vi "prius_all.vi"() -> ()   [LabVIEW 2015]
uses:
  <vilib>/Platform/TimedLoop/XDataNode/timing_clust.ctl
  <vilib>/Platform/TimedLoop/XDataNode/nitl_modes.ctl
  <vilib>/Platform/TimedLoop/XDataNode/wakeup.ctl
  <vilib>/myRIO/Instrument Drivers/Onboard IO/DIO/typedefs/DIO Reference.ctl
  <vilib>/myRIO/Common/Instrument Driver Framework/Utilities/typedefs/myRIO Generic Hardware Reference.ctl
  <vilib>/myRIO/Common/Instrument Driver Framework/Utilities/typedefs/Hardware Version Enum.ctl
  <vilib>/myRIO/Common/Instrument Driver Framework/Utilities/typedefs/myRIO v1.0 Reference.ctl
  <vilib>/myRIO/Common/Instrument Driver Framework/Utilities/typedefs/Generic FPGA Reference.ctl
  <vilib>/myRIO/Common/Instrument Driver Framework/myRIO v1.0/DIO/typedefs/DIO Channels List.ctl
  <vilib>/myRIO/Common/Instrument Driver Framework/myRIO v1.0/DIO/typedefs/DIO Channels Enum.ctl
  <vilib>/userdefined/High Color/nirio_resource_hc.ctl
  <vilib>/myRIO/Common/Instrument Driver Framework/myRIO v1.0/DIO/vis/myRIO v1.1 Open DIO.vi
  <vilib>/myRIO/Common/Instrument Driver Framework/Utilities/vis/Validate Channels.vi
  <vilib>/myRIO/Common/Instrument Driver Framework/myRIO v1.0/DIO/vis/myRIO v1.0 Reserve DIO.vi
  <vilib>/myRIO/Instrument Drivers/Onboard IO/PWM/vis/Set Duty Cycle and Frequency.vi
  <vilib>/myRIO/Common/Instrument Driver Framework/myRIO v1.0/DIO/vis/myRIO v1.0 Close DIO.vi
  <vilib>/myRIO/Common/Instrument Driver Framework/myRIO v1.0/AO/vis/myRIO v1.0 Close AO.vi
  <vilib>/myRIO/Common/Instrument Driver Framework/myRIO v1.0/PWM/vis/myRIO v1.0 Close PWM.vi
  <vilib>/myRIO/Common/Instrument Driver Framework/myRIO v1.0/Resource Manager/vis/myRIO v1.0 Reserve Channel List.vi
  <vilib>/myRIO/Common/Instrument Driver Framework/myRIO v1.0/DIO/vis/myRIO v1.0 Build MUX Configuration DIO.vi
  <vilib>/myRIO/Common/Instrument Driver Framework/myRIO v1.0/DIO/vis/myRIO v1.0 Unreserve DIO.vi
  <vilib>/myRIO/Common/Instrument Driver Framework/myRIO v1.0/AO/vis/myRIO v1.0 Unreserve AO.vi
  <vilib>/myRIO/Common/Instrument Driver Framework/myRIO v1.0/PWM/vis/myRIO v1.0 Unreserve PWM.vi
  <vilib>/myRIO/Common/Instrument Driver Framework/myRIO v1.0/Resource Manager/vis/myRIO v1.0 Reserve Channel.vi
  <vilib>/myRIO/Common/Instrument Driver Framework/myRIO v1.0/Resource Manager/vis/myRIO v1.0 Unreserve Channel.vi
  <vilib>/myRIO/Common/Instrument Driver Framework/myRIO v1.0/Resource Manager/vis/myRIO v1.0 Create Configuration List.vi
  <vilib>/myRIO/Common/Instrument Driver Framework/myRIO v1.0/Resource Manager/vis/myRIO v1.0 Unreserve Channel List.vi
  <vilib>/myRIO/Common/Instrument Driver Framework/myRIO v1.0/AO/vis/myRIO v1.0 Build MUX Configuration AO.vi
  <vilib>/myRIO/Common/Instrument Driver Framework/myRIO v1.0/PWM/vis/myRIO v1.0 Build MUX Configuration PWM.vi
  <vilib>/myRIO/Common/Instrument Driver Framework/myRIO v1.0/Resource Manager/vis/myRIO v1.0 Build Mutex Name.vi
  rio_Global.vi
  <vilib>/Utility/error.llb/Error Cluster From Error Code.vi
  <vilib>/myRIO/Common/Instrument Driver Framework/myRIO v1.0/PWM/vis/myRIO v1.0 Write PWM.vi
  <vilib>/Utility/VariantDataType/GetNumericInfo.vi
  <vilib>/myRIO/Common/Instrument Driver Framework/myRIO v1.0/myRIO v1.1 Open.vi
  <vilib>/myRIO/Common/Instrument Driver Framework/Utilities/vis/IO Manager.vi
  <vilib>/myRIO/Common/Instrument Driver Framework/Utilities/vis/Configuration Manager.vi
  <vilib>/myRIO/Common/Instrument Driver Framework/myRIO v1.0/Resource Manager/vis/myRIO v1.0 Configure IO.vi
  <vilib>/myRIO/Common/Instrument Driver Framework/myRIO v1.0/myRIO v1.0 Close.vi
  <vilib>/myRIO/Common/Instrument Driver Framework/myRIO v1.0/DIO/vis/myRIO v1.0 Write DIO.vi
  <vilib>/myRIO/Common/Instrument Driver Framework/myRIO v1.0/AO/vis/myRIO v1.0 Write AO.vi
  <vilib>/myRIO/Common/Instrument Driver Framework/myRIO v1.0/DIO/vis/myRIO v1.0 Shutdown DIO.vi
  <vilib>/myRIO/Common/Instrument Driver Framework/myRIO v1.0/PWM/vis/myRIO v1.0 Shutdown PWM.vi
  <vilib>/Analysis/Matrix/Numeric/Conversions/Array To Matrix - RA2.vi
  <vilib>/Analysis/Matrix/Numeric/Multiply/Multiply - RM,RM.vi
  <vilib>/Analysis/Matrix/Numeric/Add/Add - RM,RM.vi
  <vilib>/Analysis/baseanly.llb/Real Inverse Matrix.vi
  <vilib>/Analysis/Matrix/Numeric/Subtract/Subtract - RM,RM.vi
  <vilib>/Analysis/Matrix/Numeric/Conversions/Array To Matrix - RA.vi
  <vilib>/Analysis/Matrix/Numeric/Multiply/Multiply - R,RM.vi
  <vilib>/Analysis/Matrix/Numeric/Conversions/Matrix To Array - RM.vi
  <vilib>/myRIO/Instrument Drivers/Onboard IO/DIO/vis/myRIO DIO Open.xnode
  <vilib>/platform/TimedLoop/XDataNode/XDataNode.xnode
  <vilib>/myRIO/Instrument Drivers/Onboard IO/DIO/DIO.lvlib
  <vilib>/myRIO/Instrument Drivers/Onboard IO/PWM/PWM.lvlib
  <vilib>/myRIO/Instrument Drivers/Onboard IO/AO/AO.lvlib
  <vilib>/Analysis/Matrix/NI_Matrix.lvlib
  <vilib>/Analysis/NI_AALBase.lvlib
  <vilib>/Platform/TimedLoop/XDataNode/XDNodeRunTimeDep.lvlib
panel:
  in  "Ref_str_torque":dbl
  in  "invgain>1":dbl=4.499999999999998
  in  "mode":bool=TRUE
  in  "x":dbl
  out "Waveform Chart 2":dynamicdata(graph)=[{"t0"=timestamp(3543844041.358625 s since 1904-01-01), "dt"=1.0, "Y"=[0.015263023114702498]}, {"t0"=timestamp(3543844041.358625 s since 1904-01-01), "dt"=1.0, "Y"=[76.5]}]
  in  "x 2":dbl=0.002000000000000001 format="%#_13g"
  out "Ref_VS":dbl
  in  "y":dbl=0.003
  in  "min vel":i32=20
  in  "shift":dbl
  in  "lpf":dbl=0.8 format="%#_13g"
  in  "gain":dbl=0.79
  in  "str_gain":dbl=0.9 format="%#_13g"
  out "handle":dbl=-0.015263023114702498
  out "lane both":bool=TRUE
  out "get map name":bool
  out "map name":T1(ring)=enum."KAIST"
  in  "Steering Control":bool=TRUE
  out "fake_Ref_speed":dbl
  out "fake_Ref_str_ang":dbl
  out "Waveform Chart":dynamicdata(graph)=[{"t0"=timestamp(3543844041.358625 s since 1904-01-01), "dt"=1.0, "Y"=[0.015263023114702498]}, {"t0"=timestamp(3543844041.358625 s since 1904-01-01), "dt"=1.0, "Y"=[76.5]}]
  out "Gear":u8(ring) items=["P", "R", "N", "D"]
  out "read buffer":string="$GNGGA,114428.80,3623.46520,N,12724.00279,E,2,12,0.81,53.9,M,20.0,M,,0000*7B\r\n"
  out "yaw_rate":dbl=0.25
  out "XY Graph":cluster{"Y":dbl[], "Y":dbl[]}[](graph)=[{"Y"=[1.875, 1.875, 1.875, 1.875, 1.875, 1.875, 1.875, 1.875, 1.875, 1.875], "Y"=[0.0, 0.5, 1.0, 1.5, 2.0, 2.5, 3.0, 3.5, 4.0, 4.5]}, {"Y"=[-1.875, -1.875, -1.875, -1.875, -1.875, -1.875, -1.875, -1.875, -1.875, -1.875], "Y"=[0.0, 0.5, 1.0, 1.5, 2.0, 2.5, 3.0, 3.5, 4.0, 4.5]}, {"Y"=[-0.94, 0.94, 0.94, -0.94, -0.94], "Y"=[-3.2, -3.2, 1.5, 1.5, -3.2]}, {"Y"=[0.0, 0.0, 0.0, 0.0, 0.0, 0.0, 0.0, 0.0, 0.0, 0.0], "Y"=[0.0, 0.5, 1.0, 1.5, 2.0, 2.5, 3.0, 3.5, 4.0, 4.5]}, {"Y"=[-0.0, 0.002441079435136828, 0.009765016068527643, 0.021973905883363898, 0.03907124551911778, 0.061061937284492274, 0.08795229619902045, 0.11975005908698932, 0.15646439575426996, 0.19810592228603952, 0.2446867165104507, 0.2962203356814186, 0.3527218364413329, 0.41420779713322275, 0.48069634254055416, 0.5522071711422214, 0.6287615849803672, 0.7103825222489633, 0.7970945927225799, 0.8889241161567654, 0.9858991638044046, 1.0880496032065068, 1.1954071464308669, 1.3080054019486056, 1.4258799303560679, 1.5490683041691753, 1.677610171938241, 1.811547326954198, 1.950923780842551, 2.095785842368791, 2.246182201809347], "Y"=[0.0, 0.5, 1.0, 1.5, 2.0, 2.5, 3.0, 3.5, 4.0, 4.5, 5.0, 5.5, 6.0, 6.5, 7.0, 7.5, 8.0, 8.5, 9.0, 9.5, 10.0, 10.5, 11.0, 11.5, 12.0, 12.5, 13.0, 13.5, 14.0, 14.5, 15.0]}, {"Y"=[-0.0, 0.0008216505896712079, 0.0032866289850517205, 0.00739501506930651, 0.013146941995614725, 0.020542596208514396, 0.029582217474256822, 0.040266098919687465, 0.05259458707971021, 0.06656808195359076, 0.08218703706990027, 0.09945195956012753, 0.11836341024121566, 0.13892200370679575, 0.16112840842706078, 0.18498334685799023, 0.21048759555890229, 0.23764198531947045, 0.2664474012953235, 0.2969047831529963, 0.32901512522389, 0.3627794766672423, 0.39819894164267566, 0.4352746794916982, 0.474007904928726, 0.5143998882415417, 0.5564519555013874, 0.6001654887822383, 0.6455419263903934, 0.6925827631032746, 0.7412895504183155], "Y"=[0.0, 0.5, 1.0, 1.5, 2.0, 2.5, 3.0, 3.5, 4.0, 4.5, 5.0, 5.5, 6.0, 6.5, 7.0, 7.5, 8.0, 8.5, 9.0, 9.5, 10.0, 10.5, 11.0, 11.5, 12.0, 12.5, 13.0, 13.5, 14.0, 14.5, 15.0]}]
  out "Heading":dbl=-179.220077008385
  out "H_GPS":dbl
  out "pos":dbl[](array[numeric])=[1736.3543614568478, 3514.6262112945274]
  in  "GPS init":bool
  out "pos_gps":dbl[](array[numeric])=[42268800.0, 1.0, 1735.3231710957089, 3511.903145121578, -49.202530661854894, 42268800.0, 12.0, 18.0, 0.0, 0.81, 0.81, 0.0, 36.391086666666666, 127.4000465, 73.0] format="%#_19f"
  out "dt":dbl
  out "ecef ref":dbl[](array[numeric])=[-3119987.903302517, 4086549.99824973, 3761829.662354208]
  out "vgain":dbl=1.0353330715599283
  out "vcount":u64=227
  out "hbias":dbl=0.2579217148182668
  out "hcount":u64=1073
  out "get heading":bool
  out "get position":bool=TRUE
  out "heading error":dbl=3.127980429474107
  out "h_gps":dbl
  out "rt":dbl
  out "pos error":dbl=2.9758035193747063
  out "Kalmann init":bool
  out "VS_CAN":dbl
  out "car":refnum<k5>
  out "mdps str_ang":dbl=76.5
  out "eye":refnum<k5>
  out "APV":dbl
  out "PWM GAS":dbl=1000.0 min=1000.0 max=2000.0 step=1.0
  out "Auto":bool
  in  "Steering angle input":dbl(slide) min=-90.0 max=90.0 step=1.0 scale=-90.0..90.0
  in  "Steering angle input":bool=TRUE
  out "T init":i32=20
  out "T out":i32=20
  in  "manual speed":dbl
  in  "Velocity input":bool
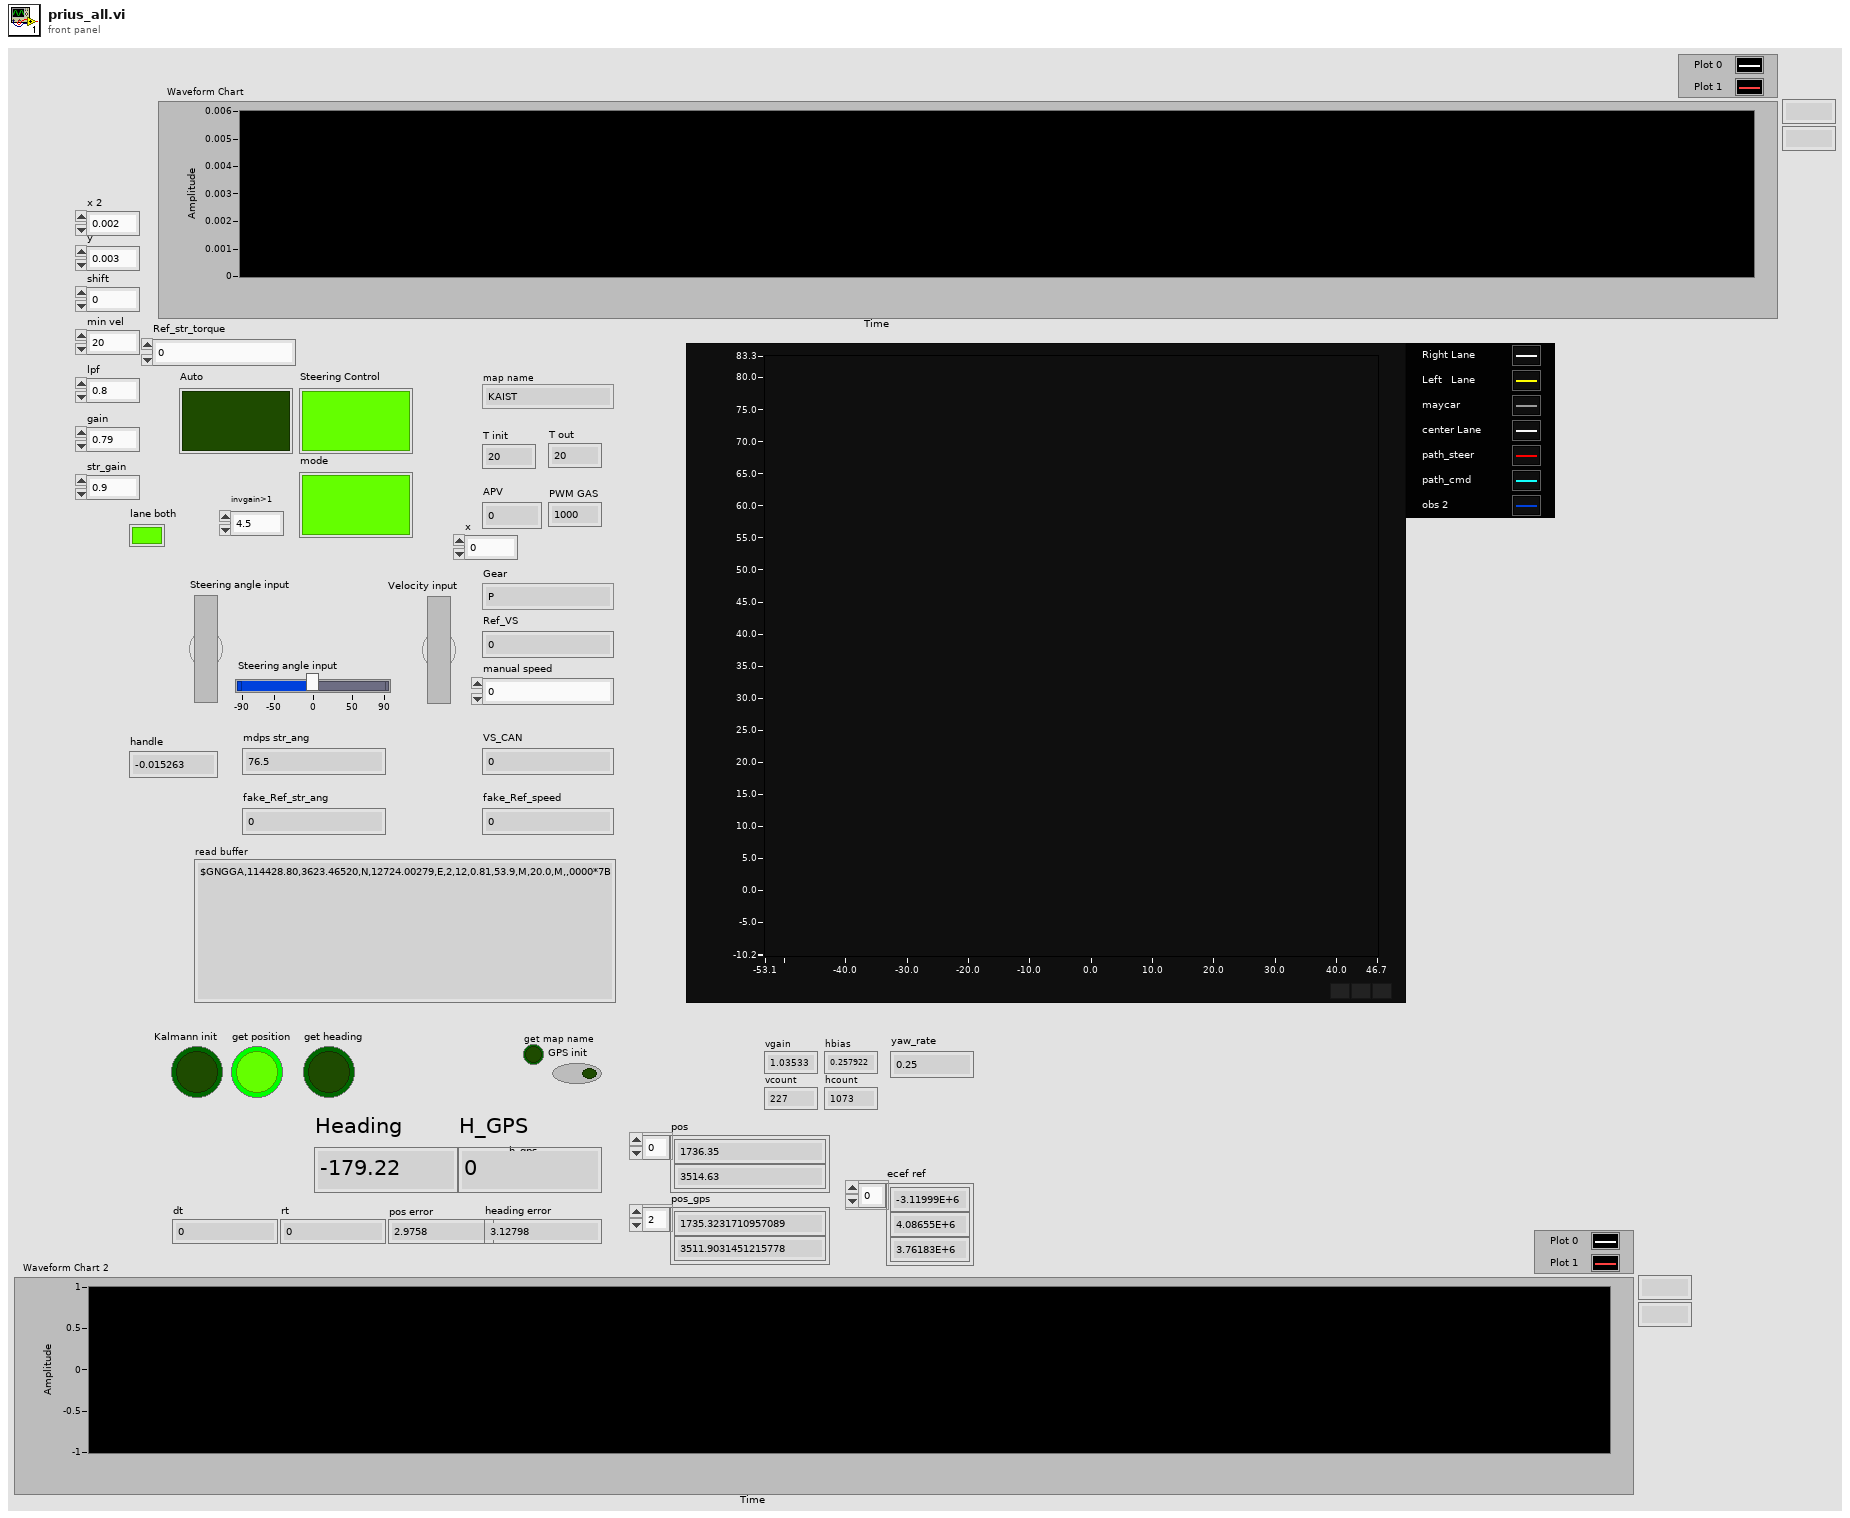
[diagram p1: front panel]
types:
  T1 = enum32{"Namyang", "Hyundai", "KAIST", "Ajou", "Munji", "Airforce", "Car", "KATRI", "Samsung", "Coex", "Gwangnaru"}
  T2 = typedef "XDNodeRunTimeDep.lvlib/timing_clust.ctl" = cluster{"Expected End [f-1]":u64, "Actual End [f-1]":u64, "Finished Late? [f-1]":bool, "Expected End [i-1]":u64, "Actual End [i-1]":u64, "Finished Late? [i-1]":bool, "Expected Start [i]":u64, "Actual Start [i]":u64, "Expected Start [f]":u64, "Actual Start [f]":u64, "Source Name":string, "Structure Name":string, "Period":i64, "Deadline":i64, "Offset":i64, "Start":i64, "Priority":i32, "Timeout":i32, "Mode":T3, "Wakeup Reason":T4, "Error":errorcluster, "Source Type":string, "Secondary Source Type":string, "Global End Time":u64, "Global Start Time":u64, "Frame Duration":u64, "Iteration Duration":u64, "Assigned CPU":i32, "I/O Scan Engine Mode":u32}
  T3 = typedef "XDNodeRunTimeDep.lvlib/nitl_modes.ctl" = enum32{"No Change", "Process missed periods, maintain original phase", "Discard missed periods, maintain original phase", "Process missed periods, ignore original phase", "Discard missed periods, ignore original phase"}
  T4 = typedef "XDNodeRunTimeDep.lvlib/wakeup.ctl" = enum32{"Normal", "Aborted", "Asynchronous wakeup", "Timing source error", "Timed loop error", "Timeout"}
  T5 = typedef "nirio_resource_hc.ctl" = tag
  T6 = typedef "Hardware Version Enum.ctl" = enum16{"Unknown", "myRIO-1900", "myRIO-1950", "roboRIO"}
  T7 = enum16{"Standard", "Buffered", "CRLF", "Immediate"}
  T8 = cluster{"identifier":u32, "timestamp":timestamp, "payload":u8[]}
  T9 = cluster{"connection ID":refnum<k16>, "net address":u32, "port":u16}
  T10 = cluster{"hash":i64, "sys time":i64, "size":i32, "data":u8[]}
  T11 = cluster{"hash":i64, "sys time":i64, "time":dbl, "yaw_rate":dbl, "mdps torque":dbl, "mdps str_ang":dbl, "VS_CAN":dbl, "lat_accel":dbl, "mcp":dbl, "accel pedal value":dbl, "tps":dbl, "odometer":dbl, "battery voltage":dbl, "WHL_SPD_RR":dbl, "WHL_SPD_RL":dbl, "WHL_SPD_FR":dbl, "WHL_SPD_FL":dbl}
  T12 = typedef "PWM.lvlib/PWM Reference.ctl" = cluster{"myRIO Reference":T13, "PWM Channels Enum":T16, "PWM Configuration":T17}
  T13 = typedef "myRIO Generic Hardware Reference.ctl" = cluster{"myRIO Model":T6, "myRIO Hardware Reference":T14}
  T14 = typedef "myRIO v1.0 Reference.ctl" = cluster{"Generic FPGA Reference":T15, "Allow multiple opens":bool}
  T15 = typedef "Generic FPGA Reference.ctl" = refnum<k20>
  T16 = typedef "PWM Channels Enum.ctl" = enum16{"Not Connected", "C/PWM0", "C/PWM1", "A/PWM0", "A/PWM1", "A/PWM2", "B/PWM0", "B/PWM1", "B/PWM2", "PWM/PWM0", "PWM/PWM1", "PWM/PWM2", "PWM/PWM3", "PWM/PWM4", "PWM/PWM5", "PWM/PWM6", "PWM/PWM7", "PWM/PWM8", "PWM/PWM9"}
  T17 = typedef "PWM.lvlib/PWM Configuration.ctl" = cluster{"Frequency":dbl, "Duty Cycle":dbl}
  T18 = typedef "AO.lvlib/AO Reference.ctl" = cluster{"myRIO Reference":T13, "AO Channel List":T19, "AO Scaling Constant List":T21}
  T19 = typedef "AO Channels List.ctl" = T20[]
  T20 = typedef "AO Channels Enum.ctl" = enum16{"Not Connected", "AudioOut/Left", "AudioOut/Right", "C/AO0", "C/AO1", "A/AO0", "A/AO1", "B/AO0", "B/AO1"}
  T21 = typedef "Analog Scaling Constants List.ctl" = T22[]
  T22 = typedef "Analog Scaling Constants.ctl" = cluster{"LSB Weight (Volts)":dbl, "Offset (Volts)":dbl, "Signed?":bool}
  T23 = typedef "DIO.lvlib/DIO Reference.ctl" = cluster{"myRIO Reference":T13, "DIO Channels List":T24}
  T24 = typedef "DIO Channels List.ctl" = T25[]
  T25 = typedef "DIO Channels Enum.ctl" = enum16{"Not Connected", "C/DIO0", "C/DIO1", "C/DIO2", "C/DIO3", "C/DIO4", "C/DIO5", "C/DIO6", "C/DIO7", "A/DIO0", "A/DIO1", "A/DIO2", "A/DIO3", "A/DIO4", "A/DIO5", "A/DIO6", "A/DIO7", "A/DIO8", "A/DIO9", "A/DIO10", "A/DIO11", "A/DIO12", "A/DIO13", "A/DIO14", "A/DIO15", "B/DIO0", "B/DIO1", "B/DIO2", "B/DIO3", "B/DIO4", "B/DIO5", "B/DIO6", "B/DIO7", "B/DIO8", "B/DIO9", "B/DIO10", "B/DIO11", "B/DIO12", "B/DIO13", "B/DIO14", "B/DIO15", "LED0", "LED1", "LED2", "LED3", "Button0", "DIO/DIO0", "DIO/DIO1", "DIO/DIO2", "DIO/DIO3", "DIO/DIO4", "DIO/DIO5", "DIO/DIO6", "DIO/DIO7", "DIO/DIO8", "DIO/DIO9", "SPI/CS0", "SPI/CS1", "SPI/CS2", "SPI/CS3", "LED RADIO (Green)", "LED RADIO (Red)", "LED COMM (Green)", "LED COMM (Red)", "LED MODE (Green)", "LED MODE (Red)"}
  T26 = cluster{"hash":i64, "sys time":i64, "ref_vel":dbl, "ref_steer":dbl, "alert":u8}
  T27 = cluster{"hash":i64, "sys time":i64, "ref_vel":dbl, "ref_steer":dbl}
  T28 = cluster{"hash":i64, "sys time":i64, "Auto":bool, "Run":bool, "Solenoid":bool, "T lim":bool, "brk_enc":u8, "B PWM":u16, "T PWM":u16, "ref_vel":dbl, "ref_bkr_enc":dbl, "ref_apv":dbl, "ref_steer":dbl}
  T29 = typedef "NI_Matrix.lvlib/RealMatrix.ctl" = dbl[][]
  T30 = cluster{"hash":i64, "sys time":i64, "dt":dbl, "x":dbl, "y":dbl, "speed":dbl, "heading":dbl, "yaw_rate":dbl}
  T31 = cluster{"Real 2D Array[0]":dbl, "Real 2D Array[1]":dbl, "Real 2D Array[2]":dbl, "Real 2D Array[3]":dbl, "Real 2D Array[4]":dbl}
  T32 = cluster{"hash":i64, "sys time":i64, "time":dbl, "x":dbl, "y":dbl, "h":dbl, "numSV":i32, "postype":i32, "lag":i32, "hordev":dbl, "lat":dbl, "lon":dbl, "hgt":dbl, "map_idx":i32}
  T33 = cluster{"output[0]":dbl, "output[1]":dbl, "output[2]":dbl, "output[3]":dbl, "output[4]":dbl, "output[5]":dbl, "output[6]":dbl, "output[7]":dbl, "output[8]":dbl, "output[9]":dbl, "output[10]":dbl, "output[11]":dbl, "output[12]":dbl, "output[13]":dbl, "output[14]":dbl}
  T34 = cluster{"hash":i64, "sys time":i64, "time":dbl, "speed":dbl, "heading":dbl, "lat":dbl, "lon":dbl}
  T35 = cluster{"output[0]":dbl, "output[1]":dbl, "output[2]":dbl, "output[3]":dbl, "output[4]":dbl, "output[5]":dbl, "output[6]":dbl}
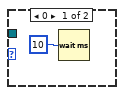
[diagram p2: hidden frame]
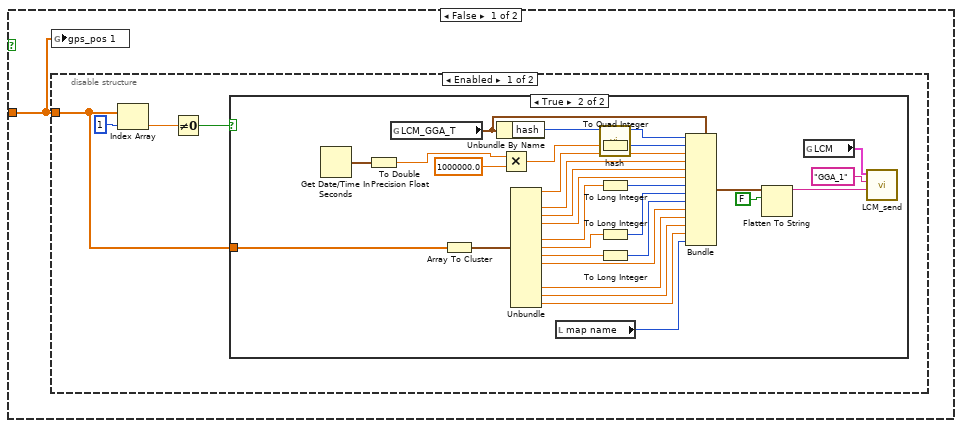
[diagram p4: hidden frame]
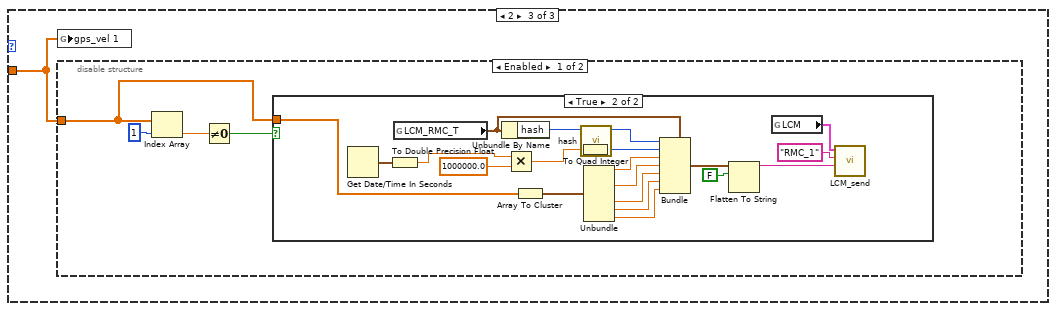
[diagram p7: hidden frame]
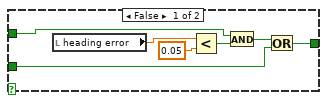
[diagram p13: hidden frame]
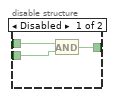
[diagram p14: hidden frame]
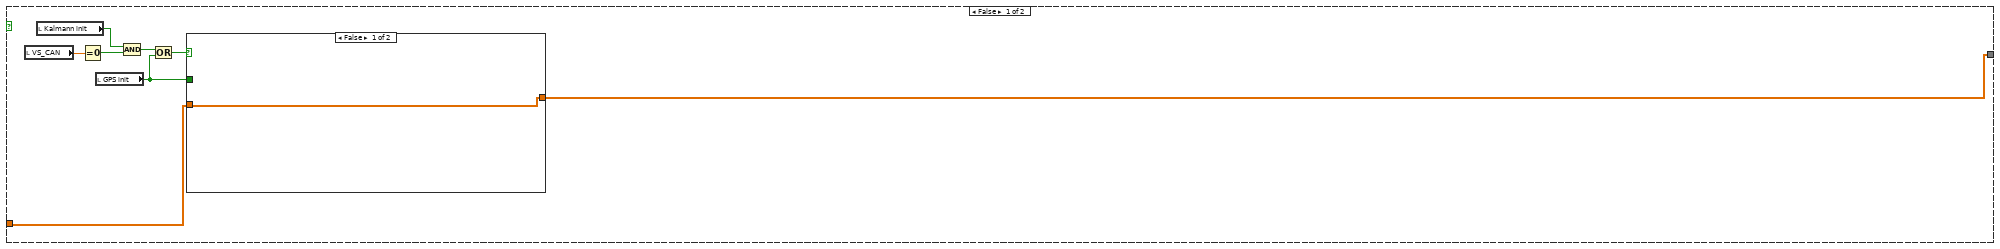
[diagram p15: hidden frame]
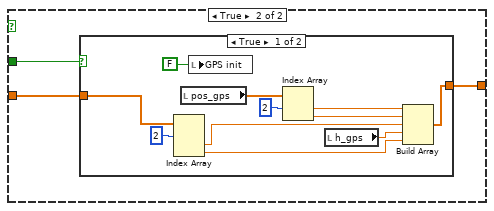
[diagram p16: hidden frame]
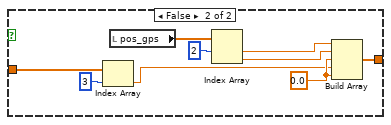
[diagram p17: hidden frame]
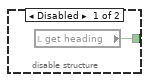
[diagram p19: hidden frame]
diagram:
  n1 = flat-sequence {
    frame #0 {
      w17 = u16 7668 ("port")
      w13 = u16 7665 ("port")
      n2 = disable-structure shown="Enabled" {
        frame Disabled {
        }
        frame Enabled {
          w36 = "Prius" ("Car_name")
          w37 = 0.0 ("Ref_str_ang")
          w38 = 1000.0 ("PWM GAS")
          w34 = FALSE ("Auto SW")
          n3 = global write "rio_Global.vi" "steering torque"(0.0 ("steering")) -> ()
          n4 = global write "rio_Global.vi" "Shift control"(0.0 ("Shift control")) -> ()
          n5 = global write "rio_Global.vi" "Solenoid"(FALSE ("CAN A 1")) -> ()
          n6 = global write "rio_Global.vi" "PWM GAS"(w38) -> ()
          n7 = global write "rio_Global.vi" "PWM Brake"(w38) -> ()
          n8 = global write "rio_Global.vi" "Ref_VS"(w37) -> ()
          n9 = global write "rio_Global.vi" "Ref_str_ang"(w37) -> ()
          n10 = global write "rio_Global.vi" "Auto"(w34) -> ()
          n11 = global write "rio_Global.vi" "Car_name"(w36) -> ()
          n12 = call "car_spec.vi"("Car_name"=w36) -> ("wheel base"=w31:dbl, "ratio"=w32:dbl, "overall width"=w33:dbl)  [unwired: 5 in, 3 out]
          n13 = global write "rio_Global.vi" "Auto SW"(w34) -> ()
          n14 = global write "rio_Global.vi" "ratio"(w32) -> ()
          n15 = global write "rio_Global.vi" "overall width"(w33) -> ()
          n16 = global write "rio_Global.vi" "wheel base"(w31) -> ()
        }
      }
      n17 = local read "eye"() -> (w19:refnum<k5>)
      n18 = local read "car"() -> (w20:refnum<k5>)
      n19 = global read "rio_Global.vi" "LCM PC"() -> (w10:T9)
      n20 = Equal?(x=refnum<k5> refnum ("connection ID"), y=w19) -> (x = y?=w21:bool)
      n21 = Equal?(x=refnum<k5> refnum ("connection ID"), y=w20) -> (x = y?=w23:bool)
      n22 = UDP Open(11:w17) -> (port=w15:refnum<k16>)  [unwired: 4 in, 2 out]
      n23 = Decrement(x=w13) -> (x-1=w12:u16)
      n24 = disable-structure shown="Enabled" {
        disable-tunnel: [w26 w29] -> w14
        disable-tunnel: w12 -> [w25 w30]
        frame Enabled {
          n25 = UDP Open(11:w25) -> (port=w26:refnum<k16>)  [unwired: 4 in, 2 out]
        }
        frame Disabled {
          n26 = String To IP(1:"239.255.76.67" ("name")) -> (0:w27:u32)
          n27 = UDP Multicast Open(10:w27, 11:w30) -> (3:w29:refnum<k16>)  [unwired: 3 in, 2 out]
        }
      }
      n28 = case shown="False" w21 {
        tunnel: w19 -> [w42 _]
        tunnel: [w41 w47] -> w18
        frame False {
          n29 = flat-sequence {
            tunnel: w42 -> [w43]
            tunnel: [w44] -> w41
            frame #0 {
              n30 = TCP Close Connection(connection ID=w43) -> ()  [unwired: 2 in, 2 out]
            }
            frame #1 {
              w45 = u16 3000  # port
              n31 = TCP Open Connection(address="192.168.0.100", remote port or service name=w45) -> (connection ID=w44:refnum<k5>)  [unwired: 3 in, 1 out]
            }
          }
        }
        frame True {
          w48 = u16 3000  # port
          n32 = TCP Open Connection(address="192.168.0.100", remote port or service name=w48) -> (connection ID=w47:refnum<k5>)  [unwired: 3 in, 1 out]
        }
      }
      "eye" <- w18
      n33 = case shown="False" w23 {
        tunnel: w20 -> [w51 _]
        tunnel: [w50 w56] -> w5
        frame False {
          n34 = flat-sequence {
            tunnel: w51 -> [w52]
            tunnel: [w53] -> w50
            frame #0 {
              n35 = TCP Close Connection(connection ID=w52) -> ()  [unwired: 2 in, 2 out]
            }
            frame #1 {
              w54 = u16 4000  # port
              n36 = TCP Open Connection(address="192.168.0.200", remote port or service name=w54) -> (connection ID=w53:refnum<k5>)  [unwired: 3 in, 1 out]
            }
          }
        }
        frame True {
          w57 = u16 4000  # port
          n37 = TCP Open Connection(address="192.168.0.200", remote port or service name=w57) -> (connection ID=w56:refnum<k5>)  [unwired: 3 in, 1 out]
        }
      }
      n38 = Bundle By Name(cluster=w10, "port"=w17, "connection ID"=w15, "net address"=u32 0) -> (w11:T9)
      n39 = global write "rio_Global.vi" "LCM PC"(w11) -> ()
      n40 = String To IP(1:"192.168.0.5" ("name")) -> (0:w2:u32)
      n41 = global read "rio_Global.vi" "LCM"() -> (w9:T9)
      n42 = Bundle By Name(cluster=w9, "port"=w13, "connection ID"=w14, "net address"=w2) -> (w8:T9)
      n43 = global write "rio_Global.vi" "LCM"(w8) -> ()
      n44 = TCP Read(connection ID=w5, bytes to read=999999, 9:1 ("timeout ms (25000)")) -> (connection ID out=→"car":refnum<k5>)  [unwired: 2 in, 2 out]
    }
    frame #1 {
      w87 = tag "B/PWM2"  # Brake
      w101 = tag[] ["B/AO0", "B/AO1"]  # Steering
      w108 = tag[] ["B/DIO4"]  # auto
      w111 = tag "B/PWM0"  # Accel
      w116 = tag[] ["B/DIO5", "B/DIO6"]  # Solenoid
      w78 = tag[] ["C/DIO7", "C/DIO6", "C/DIO5", "C/DIO0"]  # Shift X Eable
      w83 = tag[] ["C/AO0", "C/AO1"]  # Shift
      n45 = local read "eye"() -> (w92:refnum<k5>)
      n46 = local read "car"() -> (w88:refnum<k5>)
      n47 = while {
        tunnel: w92 -> [w302]
        tunnel: [w304] -> w95
        tunnel: [w303] -> w94
        shift-right: [w298] -> _
        shift-left: "" -> [w301]
        stop <- FALSE stop-if-true
        n48 = TCP Read(connection ID=w302, bytes to read=999999, 7:T7."Immediate" ("mode (standard)"), 9:1 ("timeout ms (25000)")) -> (connection ID out=w304:refnum<k5>, data out=w300:string, error out=w303:errorcluster)  [unwired: 1 in]
        n49 = Concatenate Strings(w301, w300) -> (w299:string)
        n50 = case shown="Default" w299 {
          selector: w299 -> [_ w312]
          tunnel: [_ w311] -> w298
          frame "" {
          }
          frame Default {
            n51 = flat-sequence {
              tunnel: w312 -> [w313]
              tunnel: [w314] -> w310
              tunnel: [w313] -> w309
              tunnel: [w343] -> w311
              tunnel: w310 -> [w343]
              tunnel: w309 -> [w342]
              frame #0 {
                n52 = while {
                  shift-right: [w321] -> w314
                  shift-left: w313 -> [w333]
                  stop <- w318 stop-if-true
                  w319 = "S" ("regular expression")
                  n53 = Match Pattern(string=w333, regular expression="S") -> (after substring=w331:string)  [unwired: 1 in, 3 out]
                  n54 = Match Pattern(string=w331, regular expression=" ") -> (before substring=w329:string, after substring=w326:string)  [unwired: 1 in, 2 out]
                  n55 = Hexadecimal String To Number(string=w329) -> (number=w316:u32)  [unwired: 2 in, 1 out]
                  n56 = Match Pattern(string=w326, regular expression=w319) -> (before substring=w325:string, match substring=w320:string, after substring=w322:string)  [unwired: 1 in, 1 out]
                  n57 = Not Equal?(x=w320, y=w319) -> (x != y?=w318:bool)
                  n58 = Concatenate Strings(w320, w322) -> (w321:string)
                  n59 = for {
                    N: 8 -> [_]
                    tunnel: w325 -> [w341]
                    tunnel: [w337] -> w315 mode=indexing
                    i -> [w336]
                    n60 = Multiply(x=2, y=w336) -> (x*y=w339:i32)
                    n61 = String Subset(string=w341, offset (0)=w339, length (rest)=2 ("length (rest)")) -> (substring=w334:string)
                    n62 = Hexadecimal String To Number(string=w334, default (0uL)=u8 0) -> (number=w337:u8)  [unwired: 1 in, 1 out]
                  }
                  n63 = Get Date/Time In Seconds() -> (seconds since 1Jan1904=w324:timestamp)
                  n64 = Bundle By Name(cluster=T8 {"identifier"=0, "timestamp"=timestamp(0 s since 1904-01-01), "payload"=[]} ("can cluster"), "identifier"=w316, "payload"=w315, "timestamp"=w324) -> (w323:T8)
                  n65 = call "mobileye_decoder.vi"("can cluster"=w323, "name"="Mobileye560") -> ()  [unwired: 10 in]
                }
              }
              frame #1 {
                n66 = disable-structure shown="Enabled" {
                  disable-tunnel: w342 -> [w345 _]
                  frame Enabled {
                    n67 = global read "rio_Global.vi" "LCM_CAN_RAW_SNAP"() -> (w358:T10)
                    n68 = Get Date/Time In Seconds() -> (seconds since 1Jan1904=w356:timestamp)
                    n69 = To Double Precision Float(number=w356) -> (double precision float=w355:dbl)
                    n70 = Unbundle By Name(w358) -> ("hash"=w353:i64)
                    n71 = Multiply(x=w355, y=1000000.0) -> (x*y=w357:dbl)
                    n72 = String To Byte Array(string=w345) -> (unsigned byte array=w346:u8[])
                    n73 = To Quad Integer(1:w357) -> (0:w348:i64)
                    n74 = call "hash.vi"("input"=w353) -> ("output"=w359:i64)  [unwired: 10 in]
                    n75 = Array Size(array=w346) -> (size(s)=w347:i32)
                    n76 = Bundle(cluster=w358, "hash"=w359, "sys time"=w348, "size"=w347, "data"=w346) -> (w351:T10)
                    n77 = Flatten To String(anything=w351, prepend array or string size? (T)=FALSE) -> (data string=w349:string)  [unwired: 2 in, 2 out]
                    n78 = global read "rio_Global.vi" "LCM"() -> (w350:T9)
                    n79 = call "LCM_send.vi"("DATA"=w349, "ID"="Mobileye560S", "LCM"=w350) -> ()  [unwired: 7 in, 2 out]
                  }
                  frame Disabled {
                  }
                }
              }
            }
          }
        }
      }
      n80 = while {
        tunnel: w88 -> [w209]
        tunnel: [w211] -> w89
        tunnel: [w210] -> w90
        shift-right: [w205] -> _
        shift-left: "" -> [w208]
        stop <- FALSE stop-if-true
        n81 = TCP Read(connection ID=w209, bytes to read=999999, 7:T7."Immediate" ("mode (standard)"), 9:1 ("timeout ms (25000)")) -> (connection ID out=w211:refnum<k5>, data out=w207:string, error out=w210:errorcluster)  [unwired: 1 in]
        n82 = Concatenate Strings(w208, w207) -> (w206:string)
        n83 = case shown="Default" w206 {
          selector: w206 -> [_ w219]
          tunnel: [_ w220] -> w205
          frame "" {
          }
          frame Default {
            n84 = flat-sequence {
              tunnel: w219 -> [w221]
              tunnel: [w222] -> w218
              tunnel: [w221] -> w217
              tunnel: w218 -> [w251]
              tunnel: w217 -> [w250]
              tunnel: [w251] -> w216
              tunnel: [w297] -> w220
              tunnel: w216 -> [w297]
              frame #0 {
                n85 = while {
                  shift-right: [w231] -> w222
                  shift-left: w221 -> [w241]
                  stop <- w228 stop-if-true
                  w229 = "S" ("regular expression")
                  n86 = Match Pattern(string=w241, regular expression="S") -> (after substring=w239:string)  [unwired: 1 in, 3 out]
                  n87 = Match Pattern(string=w239, regular expression=" ") -> (before substring=w237:string, after substring=w235:string)  [unwired: 1 in, 2 out]
                  n88 = Hexadecimal String To Number(string=w237) -> (number=w226:u32)  [unwired: 2 in, 1 out]
                  n89 = Match Pattern(string=w235, regular expression=w229) -> (before substring=w234:string, match substring=w230:string, after substring=w232:string)  [unwired: 1 in, 1 out]
                  n90 = Not Equal?(x=w230, y=w229) -> (x != y?=w228:bool)
                  n91 = Concatenate Strings(w230, w232) -> (w231:string)
                  n92 = for {
                    N: 8 -> [_]
                    tunnel: w234 -> [w249]
                    tunnel: [w245] -> w225 mode=indexing
                    i -> [w244]
                    n93 = Multiply(x=2, y=w244) -> (x*y=w247:i32)
                    n94 = String Subset(string=w249, offset (0)=w247, length (rest)=2 ("length (rest)")) -> (substring=w242:string)
                    n95 = Hexadecimal String To Number(string=w242, default (0uL)=u8 0) -> (number=w245:u8)  [unwired: 1 in, 1 out]
                  }
                  n96 = Get Date/Time In Seconds() -> (seconds since 1Jan1904=w233:timestamp)
                  n97 = Bundle By Name(cluster=T8 {"identifier"=0, "timestamp"=timestamp(0 s since 1904-01-01), "payload"=[]} ("can cluster"), "identifier"=w226, "payload"=w225, "timestamp"=w233) -> (w223:T8)
                  n98 = global read "rio_Global.vi" "Car_name"() -> (w224:string)
                  n99 = call "can decoder.vi"("can cluster"=w223, "name"=w224) -> ()  [unwired: 10 in]
                }
              }
              frame #1 {
                n100 = disable-structure shown="Enabled" {
                  disable-tunnel: w250 -> [w252 _]
                  frame Enabled {
                    n101 = global read "rio_Global.vi" "LCM_CAN_RAW_SNAP"() -> (w254:T10)
                    n102 = Get Date/Time In Seconds() -> (seconds since 1Jan1904=w256:timestamp)
                    n103 = To Double Precision Float(number=w256) -> (double precision float=w257:dbl)
                    n104 = Unbundle By Name(w254) -> ("hash"=w259:i64)
                    n105 = Multiply(x=w257, y=1000000.0) -> (x*y=w255:dbl)
                    n106 = String To Byte Array(string=w252) -> (unsigned byte array=w267:u8[])
                    n107 = To Quad Integer(1:w255) -> (0:w265:i64)
                    n108 = call "hash.vi"("input"=w259) -> ("output"=w253:i64)  [unwired: 10 in]
                    n109 = Array Size(array=w267) -> (size(s)=w266:i32)
                    n110 = Bundle(cluster=w254, "hash"=w253, "sys time"=w265, "size"=w266, "data"=w267) -> (w261:T10)
                    n111 = global read "rio_Global.vi" "Car_name"() -> (w264:string)
                    n112 = Flatten To String(anything=w261, prepend array or string size? (T)=FALSE) -> (data string=w263:string)  [unwired: 2 in, 2 out]
                    n113 = global read "rio_Global.vi" "LCM"() -> (w262:T9)
                    n114 = call "LCM_send.vi"("DATA"=w263, "ID"=w264, "LCM"=w262) -> ()  [unwired: 7 in, 2 out]
                  }
                  frame Disabled {
                  }
                }
              }
              frame #2 {
                n115 = Get Date/Time In Seconds() -> (seconds since 1Jan1904=w288:timestamp)
                n116 = global read "rio_Global.vi" "LCM_CAN_T"() -> (w270:T11)
                n117 = To Double Precision Float(number=w288) -> (double precision float=w289:dbl)
                n118 = global read "rio_Global.vi" "C_mdps str_ang"() -> (w269:dbl)
                n119 = global read "rio_Global.vi" "C_battery voltage"() -> (w273:dbl)
                n120 = global read "rio_Global.vi" "C_WHL_SPD_RR"() -> (w274:dbl)
                n121 = global read "rio_Global.vi" "C_WHL_SPD_RL"() -> (w275:dbl)
                n122 = global read "rio_Global.vi" "C_WHL_SPD_FR"() -> (w271:dbl)
                n123 = global read "rio_Global.vi" "C_WHL_SPD_FL"() -> (w276:dbl)
                n124 = global read "rio_Global.vi" "C_mdps torque"() -> (w283:dbl)
                n125 = Unbundle By Name(w270) -> ("hash"=w291:i64)
                n126 = Multiply(x=w289, y=1000000.0) -> (x*y=w287:dbl)
                n127 = global read "rio_Global.vi" "C_odometer"() -> (w277:dbl)
                n128 = global read "rio_Global.vi" "C_yaw_rate"() -> (w284:dbl)
                n129 = global read "rio_Global.vi" "C_VS_CAN"() -> (w282:dbl)
                n130 = global read "rio_Global.vi" "C_MCP"() -> (w280:dbl)
                n131 = global read "rio_Global.vi" "C_APV"() -> (w279:dbl)
                n132 = To Quad Integer(1:w287) -> (0:w296:i64)
                n133 = Negate(x=w269) -> (-x=w268:dbl)
                n134 = call "hash.vi"("input"=w291) -> ("output"=w286:i64)  [unwired: 10 in]
                n135 = global read "rio_Global.vi" "time"() -> (w285:dbl)
                n136 = Bundle(cluster=w270, "hash"=w286, "sys time"=w296, "time"=w285, "yaw_rate"=w284, "mdps torque"=w283, "mdps str_ang"=w268, "VS_CAN"=w282, "lat_accel"=0.0, "mcp"=w280, "accel pedal value"=w279, "tps"=0.0, "odometer"=w277, "battery voltage"=w273, "WHL_SPD_RR"=w274, "WHL_SPD_RL"=w275, "WHL_SPD_FR"=w271, "WHL_SPD_FL"=w276) -> (w293:T11)
                n137 = Flatten To String(anything=w293, prepend array or string size? (T)=FALSE) -> (data string=w295:string)  [unwired: 2 in, 2 out]
                n138 = global read "rio_Global.vi" "LCM"() -> (w294:T9)
                n139 = call "LCM_send.vi"("DATA"=w295, "ID"="CAN_T", "LCM"=w294) -> ()  [unwired: 7 in, 2 out]
              }
            }
          }
        }
      }
      n140 = call <vilib>:"Smart Open.vi"("Allow multiple opens?"=FALSE, "Channel Name"=w87) -> ("error out"=w61:errorcluster, "PWM Ref Out"=w64:T12)  [unwired: 8 in]
      n141 = call <vilib>:"Smart Open.vi"("Allow multiple opens?"=FALSE, "Channel Name"=w111) -> ("error out"=w69:errorcluster, "PWM Ref Out"=w68:T12)  [unwired: 8 in]
      n142 = call <vilib>:"Set Frequency.vi"("error in (no error)"=w61, "Frequency [Hz]"=50.0, "PWM Ref In"=w64) -> ("error out"=w60:errorcluster, "PWM Ref Out"=w63:T12)  [unwired: 6 in]
      n143 = call <vilib>:"Set Frequency.vi"("error in (no error)"=w69, "Frequency [Hz]"=50.0, "PWM Ref In"=w68) -> ("error out"=w66:errorcluster, "PWM Ref Out"=w67:T12)  [unwired: 6 in]
      n144 = call <vilib>:"Smart Open.vi"("Allow multiple opens?"=TRUE, "Channel Names"=w101) -> ("error out"=w99:errorcluster, "AO Ref Out"=w100:T18)  [unwired: 8 in]
      n145 = call <vilib>:"Smart Open.vi"("Allow multiple opens?"=FALSE, "Channel Names"=w108) -> ("error out"=w106:errorcluster, "DIO Ref Out"=w107:T23)  [unwired: 8 in]
      n146 = xnode "myRIO DIO Open.xnode"("Allow multiple opens?"=TRUE, "Channel Names"=w116) -> ("error out"=w114:errorcluster, "DIO Ref Out"=w115:T23)  [unwired: 1 in]
      n147 = xnode "myRIO DIO Open.xnode"("Allow multiple opens?"=TRUE, "Channel Names"=w78) -> ("error out"=w73:errorcluster, "DIO Ref Out"=w76:T23)  [unwired: 1 in]
      n148 = call <vilib>:"Smart Open.vi"("Allow multiple opens?"=TRUE, "Channel Names"=w83) -> ("error out"=w79:errorcluster, "AO Ref Out"=w82:T18)  [unwired: 8 in]
      n149 = node-c288(i64 10 ("Period")) -> (w72:T2)  [unwired: 3 in]
      n150 = timed-loop {
        tunnel: w115 -> [w181]
        tunnel: [w182] -> w113
        tunnel: w114 -> [w180]
        tunnel: [w176] -> w112
        tunnel: w107 -> [w174]
        tunnel: [w174] -> w105
        tunnel: w106 -> [w173]
        tunnel: [w173] -> w104
        tunnel: w100 -> [w172]
        tunnel: [w170] -> w98
        tunnel: w99 -> [w171]
        tunnel: [w169] -> w97
        tunnel: w67 -> [w178]
        tunnel: [w179] -> w110
        tunnel: w66 -> [w177]
        tunnel: [w175] -> w109
        tunnel: w63 -> [w167]
        tunnel: [w166] -> w85
        tunnel: w82 -> [w165]
        tunnel: [w164] -> w81
        tunnel: [w163] -> w80
        tunnel: w79 -> [w162]
        tunnel: w76 -> [w161]
        tunnel: [w160] -> w75
        tunnel: [w159] -> w74
        tunnel: w73 -> [w158]
        timing: w72 -> [_]
        timing-out: [_] -> w71
        tunnel: w60 -> [w128]
        tunnel: [w127] -> w59
        stop <- FALSE ("Auto") stop-if-true
        w148 = 0.0 ("y")
        n151 = node-c288() -> ()  [unwired: 1 in]
        n152 = global read "rio_Global.vi" "PWM Brake"() -> (w120:dbl)
        n153 = global read "rio_Global.vi" "PWM GAS"() -> (w123:dbl)
        n154 = global read "rio_Global.vi" "Solenoid"() -> (w121:bool)
        n155 = global read "rio_Global.vi" "steering torque"() -> (w144:dbl)
        n156 = global read "rio_Global.vi" "Shift control"() -> (w132:dbl)
        n157 = global read "rio_Global.vi" "C_VS_CAN"() -> (w140:dbl)
        n158 = global read "rio_Global.vi" "Auto"() -> (w119:bool)
        n159 = global read "rio_Global.vi" "Auto"() -> (w124:bool)
        n160 = global read "rio_Global.vi" "Auto"() -> (w122:bool)
        n161 = Select(t=w121, s=w122, f=w122) -> (s? t:f=w126:bool)
        n162 = Negate(x=w144) -> (-x=w146:dbl)
        n163 = Equal To 0?(x=w140) -> (x = 0?=w130:bool)
        n164 = Not Equal To 0?(x=w132) -> (x != 0?=w131:bool)
        n165 = Select(t=w120, s=w119, f=1000.0) -> (s? t:f=w142:dbl)
        n166 = Select(t=w123, s=w124, f=1000.0) -> (s? t:f=w147:dbl)
        n167 = global read "rio_Global.vi" "Auto"() -> (w145:bool)
        n168 = global read "rio_Global.vi" "Auto"() -> (w141:bool)
        n169 = Build Array(w126, w126) -> (w152:bool[])
        n170 = Select(t=w146, s=w145, f=w148) -> (s? t:f=w149:dbl)
        n171 = call <vilib>:"Write.vi"("error in (no error)"=w180, "Values"=w152, "DIO Ref In"=w181) -> ("error out"=w176:errorcluster, "DIO Ref Out"=w182:T23)  [unwired: 6 in]
        n172 = Compound Arithmetic op=AND(w130, w141, w131) -> (w137:bool)
        n173 = Divide(x=w142, y=20000.0) -> (x/y=w129:dbl)
        n174 = Divide(x=w147, y=20000.0) -> (x/y=w150:dbl)
        n175 = Max & Min(x=w149, y=w148) -> (min(x,y)=w154:dbl)  [unwired: 1 out]
        n176 = Select(t=w132, s=w137, f=0.0 ("element")) -> (s? t:f=w134:dbl)
        n177 = Build Array(w137, w137, w137, FALSE ("element")) -> (w139:bool[])
        n178 = call <vilib>:"Write.vi"("error in (no error)"=w158, "Values"=w139, "DIO Ref In"=w161) -> ("error out"=w159:errorcluster, "DIO Ref Out"=w160:T23)  [unwired: 6 in]
        n179 = Negate(x=w154) -> (-x=w153:dbl)
        n180 = call <vilib>:"Set Duty Cycle.vi"("error in (no error)"=w128, "Duty Cycle"=w129, "PWM Ref In"=w167) -> ("error out"=w127:errorcluster, "PWM Ref Out"=w166:T12)  [unwired: 6 in]
        n181 = call <vilib>:"Set Duty Cycle.vi"("error in (no error)"=w177, "Duty Cycle"=w150, "PWM Ref In"=w178) -> ("error out"=w175:errorcluster, "PWM Ref Out"=w179:T12)  [unwired: 6 in]
        n182 = Max & Min(x=0.0, y=w149) -> (max(x,y)=w155:dbl)  [unwired: 1 out]
        n183 = Build Array(0.0 ("element"), w134) -> (w133:dbl[])
        n184 = call <vilib>:"Write.vi"("error in (no error)"=w162, "Values"=w133, "AO Ref In"=w165) -> ("error out"=w163:errorcluster, "AO Ref Out"=w164:T18)  [unwired: 6 in]
        n185 = Build Array(w155, w153) -> (w157:dbl[])
        n186 = call <vilib>:"Write.vi"("error in (no error)"=w171, "Values"=w157, "AO Ref In"=w172) -> ("error out"=w169:errorcluster, "AO Ref Out"=w170:T18)  [unwired: 6 in]
        n187 = node-c288() -> ()  [unwired: 1 out]
      }
      n188 = node-c288(w71) -> ()  [unwired: 1 out]
      n189 = call <vilib>:"Close.vi"("error in (no error)"=w97, "AO Ref In"=w98) -> ()  [unwired: 9 in, 1 out]
      n190 = call <vilib>:"Close.vi"("error in (no error)"=w59, "PWM Ref In"=w85) -> ()  [unwired: 9 in, 1 out]
      n191 = call <vilib>:"Close.vi"("error in (no error)"=w104, "DIO Ref In"=w105) -> ()  [unwired: 9 in, 1 out]
      n192 = call <vilib>:"Close.vi"("error in (no error)"=w109, "PWM Ref In"=w110) -> ()  [unwired: 9 in, 1 out]
      n193 = call <vilib>:"Close.vi"("error in (no error)"=w112, "DIO Ref In"=w113) -> ()  [unwired: 9 in, 1 out]
      n194 = call <vilib>:"Close.vi"("error in (no error)"=w74, "DIO Ref In"=w75) -> ()  [unwired: 9 in, 1 out]
      n195 = call <vilib>:"Close.vi"("error in (no error)"=w80, "AO Ref In"=w81) -> ()  [unwired: 9 in, 1 out]
      n196 = TCP Close Connection(connection ID=w95, error in (no error)=w94) -> ()  [unwired: 1 in, 2 out]
      n197 = TCP Close Connection(connection ID=w89, error in (no error)=w90) -> ()  [unwired: 1 in, 2 out]
    }
  }
  n198 = flat-sequence {
    frame #0 {
      w380 = 0.0 ("fake_Ref_str_ang")
      w379 = FALSE ("Velocity input")
      n199 = local write "manual speed"(0.0 ("manual speed")) -> ()
      n200 = local write "Steering angle input"(0.0 ("con_vs")) -> ()
      n201 = local write "mode"(FALSE ("mode")) -> ()
      n202 = local write "Steering angle input"(FALSE ("Steering torque input")) -> ()
      n203 = global write "rio_Global.vi" "lane width"(3.5 ("lane width")) -> ()
      n204 = local write "Velocity input"(w379) -> ()
      n205 = local write "Steering Control"(w379) -> ()
      "fake_Ref_str_ang" <- w380
      "fake_Ref_speed" <- w380
      "lane both" <- FALSE ("lane both")
    }
    frame #1 {
      n206 = while {
        stop <- FALSE stop-if-true
        n207 = flat-sequence {
          tunnel: [w694] -> w384
          tunnel: w384 -> [w723]
          frame #0 {
            n208 = Wait Until Next ms Multiple(millisecond multiple=u32 10) -> ()  [unwired: 1 out]
          }
          frame #1 {
            n209 = disable-structure shown="Disabled" {
              disable-tunnel: [w390 "Mobileye" ("ID")] -> w388
              disable-tunnel: [w389 _] -> w387
              frame Enabled {
                n210 = global read "rio_Global.vi" "LCM PC"() -> (w391:T9)
                n211 = call "LCM_read.vi"("LCM"=w391) -> ("data"=w389:string, "ID"=w390:string)  [unwired: 7 in, 2 out]
              }
              frame Disabled {
              }
            }
            n212 = case shown="\"Mobileye\"" w388 {
              tunnel: w387 -> [_ _ w677]
              frame "Mobileye" {
                n213 = flat-sequence {
                  frame #0 {
                    w411 = 2 ("index")
                    w415 = 2 ("index")
                    n214 = global read "rio_Global.vi" "C_VS_CAN"() -> (w400:dbl)
                    n215 = global read "rio_Global.vi" "M_lane_right"() -> (w408:dbl[])
                    n216 = global read "rio_Global.vi" "M_headway"() -> (w394:dbl)
                    n217 = global read "rio_Global.vi" "M_lane_left"() -> (w407:dbl[])
                    n218 = Divide(x=w400, y=3.6) -> (x/y=w398:dbl)
                    n219 = Multiply(x=w398, y=w394) -> (x*y=w397:dbl)
                    n220 = Index Array(array=w407, index=w415) -> (element=w414:dbl)
                    n221 = Index Array(array=w408, index=w411) -> (element=w412:dbl)
                    n222 = Greater Or Equal?(x=w414, y=w415) -> (x >= y?=w413:bool)
                    n223 = Greater Or Equal?(x=w412, y=w411) -> (x >= y?=w410:bool)
                    n224 = Multiply(x=w397, y=2.0) -> (x*y=w396:dbl)
                    n225 = local read "lane both"() -> (w418:bool)
                    n226 = Or(x=w413, y=w410) -> (x .or. y?=w419:bool)
                    n227 = And(x=w413, y=w410) -> (x .and. y?=w417:bool)
                    n228 = Not Equal To 0?(x=w394) -> (x != 0?=w393:bool)
                    n229 = And(x=w419, y=w418) -> (x .and. y?=w416:bool)
                    n230 = Max & Min(x="x", y=w396) -> (min(x,y)=w401:dbl)  [unwired: 1 out]
                    n231 = case shown="True" w393 {
                      tunnel: w401 -> [_ w422]
                      frame False {
                      }
                      frame True {
                        n232 = global write "rio_Global.vi" "Ref_VS"(w422) -> ()
                      }
                    }
                    n233 = Or(x=w417, y=w416) -> (x .or. y?=w409:bool)
                    n234 = case shown="True" w409 {
                      tunnel: w407 -> [_ w426]
                      tunnel: w408 -> [_ w424]
                      tunnel: [_ w430] -> w420
                      frame False {
                        n235 = local write "lane both"(FALSE ("lane both")) -> ()
                      }
                      frame True {
                        w428 = 2 ("index")
                        w433 = 2 ("index")
                        n236 = Index Array(array=w426, index=w433) -> (element=w432:dbl)
                        n237 = Index Array(array=w424, index=w428) -> (element=w429:dbl)
                        n238 = Greater Or Equal?(x=w429, y=w428) -> (x >= y?=w425:bool)
                        n239 = Greater Or Equal?(x=w432, y=w433) -> (x >= y?=w427:bool)
                        n240 = And(x=w427, y=w425) -> (x .and. y?=w431:bool)
                        n241 = case shown="False" w431 {
                          tunnel: w426 -> [w455 w457]
                          tunnel: w424 -> [w450 w456]
                          tunnel: [w448 w464] -> w430
                          tunnel: w427 -> [w434 _]
                          frame False {
                            w443 = 0.2 ("y")
                            w446 = 5 ("index")
                            w454 = 5 ("index")
                            n242 = global read "rio_Global.vi" "overall width"() -> (w436:dbl)
                            n243 = Index Array(array=w455, index=w454) -> (element=w452:dbl)
                            n244 = Index Array(array=w450, index=w446) -> (element=w445:dbl)
                            n245 = global read "rio_Global.vi" "lane width"() -> (w435:dbl)
                            n246 = Multiply(x=w436, y=w443) -> (x*y=w441:dbl)
                            n247 = Add(x=w441, y=w443) -> (x+y=w437:dbl)
                            n248 = Add(x=1.0 ("y"), y=w441) -> (x+y=w438:dbl)
                            n249 = Multiply(x=w435, y=0.5) -> (x*y=w440:dbl)
                            n250 = In Range and Coerce(upper limit=w438, x=w440, lower limit=w437) -> (coerced(x)=w439:dbl)  [unwired: 1 out]
                            n251 = Add(x=w452, y=w439) -> (x+y=w451:dbl)
                            n252 = Subtract(x=w445, y=w439) -> (x-y=w444:dbl)
                            n253 = Replace Array Subset(array=w455, new element=w451, index=w454) -> (w449:dbl[])
                            n254 = Replace Array Subset(array=w450, new element=w444, index=w446) -> (w447:dbl[])
                            n255 = Select(t=w449, s=w434, f=w447) -> (s? t:f=w448:dbl[])
                          }
                          frame True {
                            n256 = Add(x=w457, y=w456) -> (x+y=w466:dbl[])
                            n257 = Index Array(array=w456, index=5) -> (element=w462:dbl)
                            n258 = Index Array(array=w457, index=5) -> (element=w459:dbl)
                            n259 = local write "lane both"(TRUE ("lane both")) -> ()
                            n260 = Subtract(x=w462, y=w459) -> (x-y=w458:dbl)
                            n261 = global write "rio_Global.vi" "lane width"(w458) -> ()
                            n262 = Multiply(x=0.5, y=w466) -> (x*y=w464:dbl[])
                          }
                        }
                      }
                    }
                    n263 = Empty Array?(array=w420) -> (empty?=w421:bool)
                    n264 = global write "rio_Global.vi" "M_lane_center"(w420) -> ()
                    n265 = case shown="False" w421 {
                      tunnel: w420 -> [w475 _]
                      tunnel: [w467 w584] -> w406
                      frame False {
                        n266 = global read "rio_Global.vi" "x_view 2"() -> (w474:dbl[])
                        n267 = disable-structure shown="Enabled" {
                          disable-tunnel: w475 -> [w497 _]
                          disable-tunnel: w474 -> [w496 w506]
                          disable-tunnel: [w495 w506] -> w472
                          frame Disabled {
                            n268 = Index Array(array=w497, index=10) -> (element=w502:dbl)
                            n269 = Multiply(x=w502, y=2.0) -> (x*y=w504:dbl)
                            n270 = Round Toward -Infinity(1:w504) -> (0:w499:dbl)
                            n271 = Max & Min(x=10.0, y=w499) -> (max(x,y)=w505:dbl)  [unwired: 1 out]
                            n272 = Array Subset(array=w496, index=0, length=w505) -> (w495:dbl[])
                          }
                          frame Enabled {
                          }
                        }
                        n273 = global read "rio_Global.vi" "C_VS_CAN"() -> (w471:dbl)
                        n274 = disable-structure shown="Enabled" {
                          disable-tunnel: w471 -> [w493 w494]
                          disable-tunnel: [w488 w494] -> w470
                          frame Disabled {
                            w489 = 32.0  # old 42
                            w490 = 15.0  # old 9
                            n275 = Subtract(x=w493, y=10.0) -> (x-y=w491:dbl)
                            n276 = In Range and Coerce(upper limit=w489, x=w491, lower limit=w490) -> (coerced(x)=w488:dbl)  [unwired: 1 out]
                          }
                          frame Enabled {
                          }
                        }
                        n277 = Index Array(array=w475, index #1=7 ("index"), index #2=6 ("index"), index #3=9 ("index"), index #4=5 ("index")) -> (element #1=w476:dbl, element #2=w483:dbl, element #3=w481:dbl, element #4=w487:dbl)
                        n278 = Square(x=w472) -> (x^2=w477:dbl[])
                        n279 = Compound Arithmetic op=MULTIPLY(w476, w472, w477) -> (w480:dbl[])
                        n280 = Compound Arithmetic op=MULTIPLY(w477, w483) -> (w479:dbl[])
                        n281 = Compound Arithmetic op=MULTIPLY(w472, w481) -> (w478:dbl[])
                        n282 = Compound Arithmetic op=ADD(w480, w479, w478, w487) -> (w473:dbl[])
                        n283 = Multiply(x=w470, y=2.0 ("y 2")) -> (x*y=w469:dbl)
                        n284 = flat-sequence {
                          tunnel: w469 -> [w527]
                          tunnel: w472 -> [w526]
                          tunnel: w473 -> [w518]
                          tunnel: [w511] -> w467
                          frame #0 {
                            n285 = disable-structure shown="Enabled" {
                              disable-tunnel: w527 -> [w545 w555]
                              disable-tunnel: w526 -> [w544 w557]
                              disable-tunnel: [w543 w560] -> w522
                              disable-tunnel: w518 -> [w533 w559]
                              frame Disabled {
                                n286 = Interpolate 1D Array(1:w545, 2:w544) -> (0:w546:dbl)
                                n287 = Interpolate 1D Array(1:w545, 2:w533) -> (0:w547:dbl)
                                n288 = Square(x=w547) -> (x^2=w536:dbl)
                                n289 = Square(x=w546) -> (x^2=w537:dbl)
                                n290 = Absolute Value(x=w547) -> (abs(x)=w535:dbl)
                                n291 = Greater Or Equal?(x=w535, y=w546) -> (x >= y?=w534:bool)
                                n292 = Add(x=w536, y=w537) -> (x+y=w538:dbl)
                                n293 = Divide(x=w538, y=w547) -> (x/y=w539:dbl)
                                n294 = Multiply(x=w539, y=0.5) -> (x*y=w541:dbl)
                                n295 = Select(t=w547, s=w534, f=w541) -> (s? t:f=w528:dbl)
                                n296 = Not A Number/Path/Refnum?(number/path/refnum=w528) -> (NaN/Path/Refnum?=w531:bool)
                                n297 = global read "rio_Global.vi" "wheel base"() -> (w532:dbl)
                                n298 = Select(t=inf, s=w531, f=w528) -> (s? t:f=w529:dbl)
                                n299 = Divide(x=w532, y=w529) -> (x/y=w542:dbl)
                                n300 = Inverse Tangent(1:w542) -> (0:w543:dbl)
                              }
                              frame Enabled {
                                n301 = Subtract(x=w555, y="min vel") -> (x-y=w553:dbl)
                                n302 = Array Subset(array=w559, index="min vel") -> (w558:dbl[])  [unwired: 1 in]
                                n303 = Array Subset(array=w557, index="min vel") -> (w556:dbl[])  [unwired: 1 in]
                                n304 = Round Toward -Infinity(1:w553) -> (0:w552:dbl)
                                n305 = Max & Min(x=1.0, y=w552) -> (max(x,y)=w551:dbl)  [unwired: 1 out]
                                n306 = for {
                                N: w551 -> [_]
                                tunnel: w556 -> [w567] mode=indexing
                                tunnel: w558 -> [w568] mode=indexing
                                tunnel: [w566] -> w549 mode=indexing
                                tunnel: [w565] -> w563 mode=indexing
                                i -> [w566]
                                n307 = Square(x=w568) -> (x^2=w576:dbl)
                                n308 = Square(x=w567) -> (x^2=w577:dbl)
                                n309 = Absolute Value(x=w568) -> (abs(x)=w575:dbl)
                                n310 = Greater Or Equal?(x=w575, y=w567) -> (x >= y?=w574:bool)
                                n311 = Add(x=w576, y=w577) -> (x+y=w578:dbl)
                                n312 = Divide(x=w578, y=w568) -> (x/y=w579:dbl)
                                n313 = Multiply(x=w579, y=0.5) -> (x*y=w581:dbl)
                                n314 = Select(t=w568, s=w574, f=w581) -> (s? t:f=w569:dbl)
                                n315 = Not A Number/Path/Refnum?(number/path/refnum=w569) -> (NaN/Path/Refnum?=w572:bool)
                                n316 = global read "rio_Global.vi" "wheel base"() -> (w573:dbl)
                                n317 = Select(t=inf, s=w572, f=w569) -> (s? t:f=w570:dbl)
                                n318 = Divide(x=w573, y=w570) -> (x/y=w582:dbl)
                                n319 = Inverse Tangent(1:w582) -> (0:w565:dbl)
                                }
                                n320 = Increment(x=w549) -> (x+1=w548:i32[])
                                n321 = Add Array Elements(numeric array=w548) -> (sum=w564:i32)
                                n322 = Divide(x=w548, y=w564) -> (x/y=w562:dbl[])
                                n323 = Multiply(x=w563, y=w562) -> (x*y=w561:dbl[])
                                n324 = Add Array Elements(numeric array=w561) -> (sum=w560:dbl)
                              }
                            }
                            n325 = Multiply(x=180.0 ("y"), y=w522) -> (x*y=w523:dbl)
                            n326 = Divide(x=w523, y=3.141592653589793) -> (x/y=w525:dbl)
                            n327 = global read "rio_Global.vi" "ratio"() -> (w510:dbl)
                            n328 = Multiply(x=w510, y=w525) -> (x*y=w509:dbl)
                            n329 = Multiply(x=w509, y=1.0 ("y 3")) -> (x*y=w508:dbl)
                            n330 = Negate(x=w508) -> (-x=w519:dbl)
                            n331 = local read "handle"() -> (w517:dbl)
                            n332 = Not A Number/Path/Refnum?(number/path/refnum=w519) -> (NaN/Path/Refnum?=w520:bool)
                            n333 = Multiply(x=w517, y="str_gain") -> (x*y=w513:dbl)
                            n334 = Decrement(x="str_gain") -> (x-1=w515:dbl)
                            n335 = Select(t=w517, s=w520, f=w519) -> (s? t:f=w514:dbl)
                            n336 = Multiply(x=w515, y=w514) -> (x*y=w512:dbl)
                            n337 = Subtract(x=w513, y=w512) -> (x-y=w511:dbl)
                          }
                        }
                      }
                      frame True {
                        n338 = local read "handle"() -> (w585:dbl)
                        n339 = Multiply(x=w585, y=0.995) -> (x*y=w584:dbl)
                      }
                    }
                    "handle" <- w406
                    n340 = Negate(x=w406) -> (-x=w404:dbl)
                    n341 = Multiply(x=w404, y="gain") -> (x*y=w403:dbl)
                    n342 = global write "rio_Global.vi" "Ref_str_ang"(w403) -> ()
                  }
                  frame #1 {
                    w592 = 2 ("index")
                    w595 = 2 ("index")
                    n343 = global read "rio_Global.vi" "M_lane_right"() -> (w587:dbl[])
                    n344 = global read "rio_Global.vi" "M_lane_left"() -> (w588:dbl[])
                    n345 = Index Array(array=w588, index=w595) -> (element=w594:dbl)
                    n346 = Index Array(array=w587, index=w592) -> (element=w593:dbl)
                    n347 = Greater Or Equal?(x=w594, y=w595) -> (x >= y?=w589:bool)
                    n348 = Greater Or Equal?(x=w593, y=w592) -> (x >= y?=w590:bool)
                    n349 = Or(x=w589, y=w590) -> (x .or. y?=w591:bool)
                    n350 = case shown="True" w591 {
                      tunnel: w590 -> [_ w623]
                      tunnel: [w596 w612] -> w586
                      tunnel: w589 -> [_ w626]
                      tunnel: w588 -> [_ w617]
                      tunnel: w587 -> [_ w616]
                      frame False {
                        n351 = global read "rio_Global.vi" "Ref_str_torque"() -> (w597:dbl)
                        n352 = Multiply(x=w597, y=0.997) -> (x*y=w596:dbl)
                      }
                      frame True {
                        n353 = disable-structure shown="Enabled" {
                          disable-tunnel: [w631 w634] -> w622
                          disable-tunnel: [w630 w656] -> w620
                          disable-tunnel: w617 -> [w629 w665]
                          disable-tunnel: w616 -> [w628 w635]
                          frame Disabled {
                            n354 = Index Array(array=w629, index=5) -> (element=w630:dbl)
                            n355 = Index Array(array=w628, index=5) -> (element=w631:dbl)
                          }
                          frame Enabled {
                            n356 = global read "rio_Global.vi" "C_VS_CAN"() -> (w664:dbl)
                            n357 = global read "rio_Global.vi" "C_VS_CAN"() -> (w640:dbl)
                            n358 = In Range and Coerce(upper limit=45.0, x=w664, lower limit=15.0) -> (coerced(x)=w653:dbl)  [unwired: 1 out]
                            n359 = In Range and Coerce(upper limit=45.0, x=w640, lower limit=15.0) -> (coerced(x)=w650:dbl)  [unwired: 1 out]
                            n360 = Index Array(array=w665, index #1=7 ("index"), index #2=6 ("index"), index #3=9 ("index"), index #4=5 ("index")) -> (element #1=w661:dbl, element #2=w654:dbl, element #3=w652:dbl, element #4=w657:dbl)
                            n361 = Index Array(array=w635, index #1=7 ("index"), index #2=6 ("index"), index #3=9 ("index"), index #4=5 ("index")) -> (element #1=w643:dbl, element #2=w649:dbl, element #3=w651:dbl, element #4=w647:dbl)
                            n362 = Square(x=w653) -> (x^2=w655:dbl)
                            n363 = Square(x=w650) -> (x^2=w648:dbl)
                            n364 = Multiply(x=w655, y=w654) -> (x*y=w659:dbl)
                            n365 = Multiply(x=w653, y=w652) -> (x*y=w658:dbl)
                            n366 = Multiply(x=w648, y=w649) -> (x*y=w645:dbl)
                            n367 = Multiply(x=w650, y=w651) -> (x*y=w646:dbl)
                            n368 = Compound Arithmetic op=MULTIPLY(w661, w655, w653) -> (w660:dbl)
                            n369 = Compound Arithmetic op=MULTIPLY(w643, w648, w650) -> (w644:dbl)
                            n370 = Compound Arithmetic op=ADD(w660, w659, w658, w657) -> (w656:dbl)
                            n371 = Compound Arithmetic op=ADD(w644, w645, w646, w647) -> (w634:dbl)
                          }
                        }
                        n372 = global read "rio_Global.vi" "C_VS_CAN"() -> (w615:dbl)
                        n373 = Square(x=w615) -> (x^2=w614:dbl)
                        n374 = global read "rio_Global.vi" "lane width"() -> (w619:dbl)
                        n375 = Divide(x=w614, y=-28800.0) -> (x/y=w611:dbl)
                        n376 = Subtract(x=w622, y=w619) -> (x-y=w624:dbl)
                        n377 = Add(x=w620, y=w619) -> (x+y=w618:dbl)
                        n378 = global read "rio_Global.vi" "C_Right light"() -> (w603:bool)
                        n379 = Multiply(x=w611, y="invgain>1") -> (x*y=w610:dbl)
                        n380 = Select(t=w620, s=w626, f=w624) -> (s? t:f=w625:dbl)
                        n381 = Select(t=w622, s=w623, f=w618) -> (s? t:f=w621:dbl)
                        n382 = global read "rio_Global.vi" "C_Left light"() -> (w601:bool)
                        n383 = Negate(x=w625) -> (-x=w627:dbl)
                        n384 = Exponential(1:w610) -> (0:w607:dbl)
                        n385 = Subtract(x=w627, y=w621) -> (x-y=w600:dbl)
                        n386 = Exclusive Or(1:w603, 2:w601) -> (0:w602:bool)
                        n387 = Multiply(x=w607, y=0.125) -> (x*y=w606:dbl)
                        n388 = case shown="True" w602 {
                          tunnel: w601 -> [_ w676]
                          tunnel: [w670 w671] -> w599
                          tunnel: w600 -> [w670 w673]
                          frame False {
                          }
                          frame True {
                            n389 = Select(t=1.0, s=w676, f=-1.0) -> (s? t:f=w672:dbl)
                            n390 = Add(x=w673, y=w672) -> (x+y=w671:dbl)
                          }
                        }
                        n391 = Max & Min(x=w606, y=0.01) -> (max(x,y)=w605:dbl)  [unwired: 1 out]
                        n392 = Multiply(x=w599, y=w605) -> (x*y=w612:dbl)
                      }
                    }
                    n393 = global write "rio_Global.vi" "Ref_str_torque"(w586) -> ()
                  }
                }
              }
              frame Default {
              }
              frame "CON_INPUT_T" {
                n394 = global read "rio_Global.vi" "CON_INPUT_T 2"() -> (w679:T26)
                n395 = Unflatten From String(type=w679, binary string=w677, data includes array or string size? (T)=FALSE) -> (value=w678:T26, error out=w680:errorcluster)  [unwired: 2 in, 1 out]
                n396 = case shown="Error" w680 {
                  tunnel: w678 -> [w685 _]
                  tunnel: w677 -> [_ w692]
                  frame No Error {
                    n397 = Unbundle By Name(w685) -> ("ref_vel"=w684:dbl, "ref_steer"=w683:dbl)
                    n398 = global write "rio_Global.vi" "Ref_VS"(w684) -> ()
                    n399 = Negate(x=w683) -> (-x=w682:dbl)
                    n400 = global write "rio_Global.vi" "Ref_str_ang"(w682) -> ()
                  }
                  frame Error {
                    n401 = global read "rio_Global.vi" "CON_INPUT_T"() -> (w690:T27)
                    n402 = Unflatten From String(type=w690, binary string=w692, data includes array or string size? (T)=FALSE) -> (value=w686:T27)  [unwired: 2 in, 2 out]
                    n403 = Unbundle By Name(w686) -> ("ref_vel"=w689:dbl, "ref_steer"=w688:dbl)
                    n404 = Negate(x=w688) -> (-x=w687:dbl)
                    n405 = global write "rio_Global.vi" "Ref_VS"(w689) -> ()
                    n406 = global write "rio_Global.vi" "Ref_str_ang"(w687) -> ()
                  }
                }
              }
            }
          }
          frame #2 {
            n407 = global read "rio_Global.vi" "Ref_VS"() -> (w702:dbl)
            n408 = global read "rio_Global.vi" "C_gear selector disp"() -> (w695:u8)
            "Gear" <- w695
            n409 = Select(t=w702, s="Velocity input", f="manual speed") -> (s? t:f=w699:dbl)
            n410 = Sign(1:w699) -> (0:w698:dbl)
            n411 = To Long Integer(number=w698) -> (32bit integer=w697:i32)
            n412 = case shown="1" w697 {
              tunnel: [w704 _ w710] -> w696
              tunnel: w695 -> [w707 _ w713]
              frame -1 {
                n413 = Not Equal?(x=w707, y=u8 1) -> (x != y?=w706:bool)
                n414 = Select(t=-2.0 ("element"), s=w706, f=0.0) -> (s? t:f=w704:dbl)
              }
              frame 0, Default {
              }
              frame 1 {
                n415 = Not Equal?(x=w713, y=u8 3) -> (x != y?=w711:bool)
                n416 = Select(t=2.0 ("element"), s=w711, f=0.0) -> (s? t:f=w710:dbl)
              }
            }
            n417 = case shown="3" w695 {
              tunnel: [_ w715 w720] -> w694
              tunnel: w699 -> [_ w717 w721]
              frame 0, Default {
                # "P,N"
              }
              frame 3 {
                # "D"
                n418 = Greater Than 0?(x=w717) -> (x > 0?=w718:bool)
                n419 = Select(t=w717, s=w718, f=0.0) -> (s? t:f=w715:dbl)
              }
              frame 1 {
                # "R"
                n420 = Less Than 0?(x=w721) -> (x < 0?=w722:bool)
                n421 = Select(t=w721, s=w722, f=0.0) -> (s? t:f=w720:dbl)
              }
            }
            "Ref_VS" <- w694
            n422 = global read "rio_Global.vi" "C_APV"() -> (→"APV":dbl)
            n423 = global write "rio_Global.vi" "Shift control"(w696) -> ()
          }
          frame #3 {
            n424 = global read "rio_Global.vi" "C_VS_CAN"() -> (w725:dbl)
            n425 = global read "rio_Global.vi" "C_VS_CAN"() -> (w727:dbl)
            n426 = global read "rio_Global.vi" "C_MCP"() -> (w732:dbl)
            n427 = feedback #1(w725) -> (w724:dbl)
            n428 = feedback-in #1(w725) -> ()
            n429 = Subtract(x=w723, y=w727) -> (x-y=w726:dbl)
            n430 = Less?(x=w732, y=5.0) -> (x < y?=w731:bool)
            n431 = case shown="True" w731 {
              tunnel: w723 -> [_ w794]
              tunnel: [_ w781] -> w739
              tunnel: w725 -> [_ w780]
              tunnel: w724 -> [_ w779]
              frame False {
              }
              frame True {
                w786 = 0.09999999999999998 ("lpf gain speed")
                n432 = Subtract(x=w780, y=w779) -> (x-y=w790:dbl)
                n433 = Multiply(x=w790, y=5.0) -> (x*y=w789:dbl)
                n434 = Add(x=w780, y=w789) -> (x+y=w788:dbl)
                n435 = Subtract(x=w794, y=w788) -> (x-y=w793:dbl)
                n436 = local read "fake_Ref_speed"() -> (w785:dbl)
                n437 = Decrement(x=w786) -> (x-1=w784:dbl)
                n438 = Multiply(x=45.0 ("x 2"), y=w793) -> (x*y=w787:dbl)
                n439 = Multiply(x=w787, y=w786) -> (x*y=w783:dbl)
                n440 = Multiply(x=w784, y=w785) -> (x*y=w782:dbl)
                n441 = Subtract(x=w783, y=w782) -> (x-y=w781:dbl)
              }
            }
            n442 = Less?(x=w726, y=-2.0 ("lower limit")) -> (x < y?=w729:bool)
            n443 = case shown="True" w729 {
              tunnel: [w746 w768] -> w728
              tunnel: w723 -> [w750 w769]
              tunnel: w726 -> [w752 w760]
              frame False {
                n444 = global read "rio_Global.vi" "PWM Brake"() -> (w759:dbl)
                n445 = Greater?(x=w752, y=1.0) -> (0:w755:bool)
                n446 = Equal To 0?(x=w750) -> (x = 0?=w749:bool)
                n447 = Multiply(x=w759, y=0.999) -> (x*y=w757:dbl)
                n448 = Max & Min(x=w757, y=1000.0) -> (max(x,y)=w753:dbl)  [unwired: 1 out]
                n449 = Select(t=1000.0, s=w755, f=w753) -> (s? t:f=w747:dbl)
                n450 = Select(t=2000.0, s=w749, f=w747) -> (s? t:f=w746:dbl)
              }
              frame True {
                w766 = 0.5 ("gain brake")
                w775 = 10.0 ("y")
                n451 = Absolute Value(x=w760) -> (abs(x)=w777:dbl)
                n452 = Add(x=w777, y=w775) -> (x+y=w776:dbl)
                n453 = Multiply(x=w776, y=w775) -> (x*y=w774:dbl)
                n454 = Threshold 1D Array(2:w774, 3:dbl[] [10.0, 15.0, 25.0, 50.0, 80.0, 120.0, 170.0, 230.0, 290.0, 350.0, 420.0]) -> (0:w772:dbl)  [unwired: 1 in]
                n455 = global read "rio_Global.vi" "PWM Brake"() -> (w764:dbl)
                n456 = Interpolate 1D Array(1:w772, 2:dbl[] [1000.0, 1100.0, 1200.0, 1300.0, 1400.0, 1500.0, 1600.0, 1700.0, 1800.0, 1900.0, 2000.0]) -> (0:w767:dbl)
                n457 = Decrement(x=w766) -> (x-1=w765:dbl)
                n458 = Multiply(x=w767, y=w766) -> (x*y=w762:dbl)
                n459 = Multiply(x=w765, y=w764) -> (x*y=w763:dbl)
                n460 = Subtract(x=w762, y=w763) -> (x-y=w761:dbl)
                n461 = Equal To 0?(x=w769) -> (x = 0?=w770:bool)
                n462 = Select(t=2000.0, s=w770, f=w761) -> (s? t:f=w768:dbl)
              }
            }
            n463 = global read "rio_Global.vi" "C_MCP"() -> (w738:dbl)
            n464 = global read "rio_Global.vi" "Auto"() -> (w735:bool)
            "Auto" <- w735
            n465 = local read "T out"() -> (w741:i32)
            n466 = local read "T init"() -> (w740:i32)
            n467 = Greater Or Equal?(x=w740, y=w741) -> (x >= y?=w736:bool)
            n468 = Less?(x=w738, y=5.0) -> (x < y?=w743:bool)
            n469 = Compound Arithmetic op=AND(w735, w743, w736) -> (w742:bool)
            n470 = local write "fake_Ref_speed"(w739) -> ()
            n471 = case shown="True" w742 {
              tunnel: [1000.0 ("Numeric") w810] -> w734
              tunnel: w739 -> [_ w805]
              tunnel: w741 -> [w795 _]
              tunnel: [_ TRUE] -> w737
              frame False {
                n472 = local read "T init"() -> (w796:i32)
                n473 = Less Or Equal?(x=w796, y=w795) -> (x <= y?=w797:bool)
                n474 = case shown="True" w797 {
                  tunnel: w795 -> [_ w800]
                  frame False {
                    n475 = local write "T init"(1 ("T init")) -> ()
                  }
                  frame True {
                    n476 = local read "T init"() -> (w803:i32)
                    n477 = Increment(x=w803) -> (x+1=w802:i32)
                    n478 = Max & Min(x=w802, y=w800) -> (min(x,y)=w801:i32)  [unwired: 1 out]
                    n479 = local write "T init"(w801) -> ()
                  }
                }
              }
              frame True {
                w809 = 1000.0 ("x")
                n480 = Add(x=w805, y=1000.0 ("PWM GAS")) -> (x+y=w812:dbl)
                n481 = In Range and Coerce(upper limit=1700.0, x=w812, lower limit=w809) -> (coerced(x)=w810:dbl)  [unwired: 1 out]
                n482 = Subtract(x=w810, y=w809) -> (x-y=w808:dbl)
                n483 = Multiply(x=w808, y=0.1) -> (x*y=w806:dbl)
                n484 = To Long Integer(number=w806) -> (32bit integer=w815:i32)
                n485 = Add(x=w815, y=20) -> (x+y=w817:i32)
                "T out" <- w817
                n486 = Increment(x=w817) -> (x+1=→"T init":i32)
              }
            }
            "PWM GAS" <- w734
            n487 = disable-structure shown="Enabled" {
              disable-tunnel: w728 -> [w745 _]
              frame Enabled {
                n488 = global write "rio_Global.vi" "PWM Brake"(w745) -> ()
              }
              frame Disabled {
              }
            }
            n489 = global write "rio_Global.vi" "Solenoid"(w737) -> ()
            n490 = global write "rio_Global.vi" "PWM GAS"(w734) -> ()
          }
          frame #4 {
            n491 = disable-structure shown="Disabled" {
              disable-tunnel: [w828 TRUE] -> w826
              frame Disabled {
                n492 = global read "rio_Global.vi" "C_Right light"() -> (w829:bool)
                n493 = global read "rio_Global.vi" "C_Left light"() -> (w830:bool)
                n494 = Not Or(1:w829, 2:w830) -> (0:w828:bool)
              }
              frame Enabled {
              }
            }
            n495 = global read "rio_Global.vi" "C_mdps str_ang"() -> (w827:dbl)
            n496 = And(x="Steering Control", y=w826) -> (x .and. y?=w824:bool)
            n497 = case shown="True" w824 {
              tunnel: [w832 w846] -> w820
              tunnel: w827 -> [_ w868]
              frame False {
                n498 = local write "fake_Ref_str_ang"(0.0 ("Manual Steering angle")) -> ()
                n499 = global read "rio_Global.vi" "steering torque"() -> (w834:dbl)
                n500 = Multiply(x=w834, y=0.9) -> (x*y=w832:dbl)
              }
              frame True {
                n501 = global read "rio_Global.vi" "Ref_str_ang"() -> (w871:dbl)
                n502 = Select(t=w871, s="Steering angle input", f="Steering angle input") -> (s? t:f=w845:dbl)
                n503 = Add(x=w845, y="shift") -> (x+y=w843:dbl)
                n504 = Subtract(x=w843, y=w868) -> (x-y=w853:dbl)
                n505 = global write "rio_Global.vi" "cmd steer"(w843) -> ()
                n506 = disable-structure shown="Enabled" {
                  disable-tunnel: w853 -> [w877 w881]
                  disable-tunnel: [w875 w881] -> w852
                  frame Enabled {
                    n507 = Absolute Value(x=w877) -> (abs(x)=w880:dbl)
                    n508 = Greater?(x=w880, y=0.001) -> (0:w878:bool)
                    n509 = Select(t=w877, s=w878, f=0.0) -> (s? t:f=w875:dbl)
                  }
                  frame Disabled {
                  }
                }
                n510 = Absolute Value(x=w852) -> (abs(x)=w862:dbl)
                n511 = Sign(1:w852) -> (0:w859:dbl)
                n512 = Multiply(x="x 2", y=w862) -> (x*y=w861:dbl)
                n513 = Square Root(x=w861) -> (sqrt(x)=w860:dbl)
                n514 = Multiply(x=w860, y=w859) -> (x*y=w858:dbl)
                n515 = In Range and Coerce(upper limit=0.4, x=w858, lower limit=-0.4) -> (coerced(x)=w863:dbl, In Range?=w864:bool)
                n516 = case shown="True" w864 {
                  tunnel: w852 -> [_ w886]
                  tunnel: [_ w883] -> w855
                  frame False {
                  }
                  frame True {
                    n517 = Sign(1:w886) -> (0:w885:dbl)
                    n518 = local read "fake_Ref_str_ang"() -> (w887:dbl)
                    n519 = Multiply(x=w885, y="y") -> (x*y=w884:dbl)
                    n520 = Add(x=w887, y=w884) -> (x+y=w883:dbl)
                  }
                }
                n521 = disable-structure shown="Enabled" {
                  disable-tunnel: [w872 "Ref_str_torque"] -> w837
                  frame Enabled {
                    n522 = global read "rio_Global.vi" "Ref_str_torque"() -> (w873:dbl)
                    n523 = Negate(x=w873) -> (-x=w872:dbl)
                  }
                  frame Disabled {
                  }
                }
                n524 = In Range and Coerce(upper limit=0.4, x=w855, lower limit=-0.4) -> (coerced(x)=w854:dbl)  [unwired: 1 out]
                n525 = global read "rio_Global.vi" "steering torque"() -> (w851:dbl)
                n526 = In Range and Coerce(upper limit=0.4, x=w837, lower limit=-0.4) -> (coerced(x)=w836:dbl)  [unwired: 1 out]
                n527 = Add(x=w863, y=w854) -> (x+y=w841:dbl)
                n528 = local write "fake_Ref_str_ang"(w854) -> ()
                n529 = Multiply(x=w851, y="lpf") -> (x*y=w847:dbl)
                n530 = Decrement(x="lpf") -> (x-1=w849:dbl)
                n531 = Select(t=w841, s="mode", f=w836) -> (s? t:f=w840:dbl)
                n532 = Multiply(x=w849, y=w840) -> (x*y=w848:dbl)
                n533 = Subtract(x=w847, y=w848) -> (x-y=w846:dbl)
              }
            }
            n534 = Add(x=w820, y=-0.031 ("y 2")) -> (x+y=w819:dbl)
            n535 = global read "rio_Global.vi" "Auto"() -> (w823:bool)
            n536 = Select(t=w819, s=w823, f=0.0) -> (s? t:f=w821:dbl)
            n537 = global write "rio_Global.vi" "steering torque"(w821) -> ()
          }
          frame #5 {
            n538 = global read "rio_Global.vi" "Auto"() -> (w915:bool)
            n539 = Get Date/Time In Seconds() -> (seconds since 1Jan1904=w905:timestamp)
            n540 = global read "rio_Global.vi" "C_mdps str_ang"() -> (→"mdps str_ang":dbl)
            n541 = global read "rio_Global.vi" "steering torque"() -> (w914:dbl)
            n542 = global read "rio_Global.vi" "Ref_str_torque"() -> (w889:dbl)
            n543 = global read "rio_Global.vi" "LCM_CON_T"() -> (w901:T28)
            n544 = To Double Precision Float(number=w905) -> (double precision float=w906:dbl)
            n545 = case shown="False" w915 {
              frame False {
                w919 = 0.0 ("Manual Steering angle")
                n546 = local write "fake_Ref_str_ang"(w919) -> ()
                n547 = local write "fake_Ref_speed"(w919) -> ()
              }
              frame True {
              }
            }
            n548 = Negate(x=w889) -> (-x=w888:dbl)
            n549 = global read "rio_Global.vi" "cmd steer"() -> (w891:dbl)
            n550 = Unbundle By Name(w901) -> ("hash"=w908:i64)
            n551 = Multiply(x=w906, y=1000000.0) -> (x*y=w904:dbl)
            n552 = Build Array(w888, w914) -> (w917:dbl[])
            n553 = global read "rio_Global.vi" "PWM Brake"() -> (w897:dbl)
            n554 = global read "rio_Global.vi" "PWM GAS"() -> (w896:dbl)
            n555 = global read "rio_Global.vi" "Solenoid"() -> (w898:bool)
            n556 = To Quad Integer(1:w904) -> (0:w913:i64)
            n557 = Negate(x=w891) -> (-x=w890:dbl)
            n558 = call "hash.vi"("input"=w908) -> ("output"=w903:i64)  [unwired: 10 in]
            n559 = call "Convert to Dynamic Data"("Array"=w917) -> ("Dynamic Data Type"=→"Waveform Chart":dynamicdata)  [unwired: 3 in]
            n560 = local read "Ref_VS"() -> (w895:dbl)
            n561 = global read "rio_Global.vi" "Auto"() -> (w900:bool)
            n562 = Bundle(cluster=w901, "hash"=w903, "sys time"=w913, "Auto"=w900, "Run"=w900, "Solenoid"=w898, "T lim"=FALSE, "brk_enc"=u8 0, "B PWM"=w897, "T PWM"=w896, "ref_vel"=w895, "ref_bkr_enc"=0.0, "ref_apv"=0.0, "ref_steer"=w890) -> (w910:T28)
            n563 = Flatten To String(anything=w910, prepend array or string size? (T)=FALSE) -> (data string=w912:string)  [unwired: 2 in, 2 out]
            n564 = global read "rio_Global.vi" "LCM"() -> (w911:T9)
            n565 = call "LCM_send.vi"("DATA"=w912, "ID"="CON_T", "LCM"=w911) -> ()  [unwired: 7 in, 2 out]
          }
        }
      }
    }
  }
  n566 = disable-structure shown="Enabled" {
    frame Enabled {
      n567 = flat-sequence {
        tunnel: [dbl[] [0.0, 0.0, 0.0, 0.0, 0.0] ("pos(i)")] -> w920
        tunnel: w920 -> [w935]
        frame #0 {
          w927 = u64 1
          w924 = 0.0 ("dh_hat")
          n568 = local write "GPS init"(FALSE ("get heading")) -> ()
          n569 = call "getecefdcmref.vi"("map name"=T1."KATRI") -> ("XYZ"=w922:dbl[])  [unwired: 10 in, 4 out]
          n570 = local write "ecef ref"(w922) -> ()
          "vgain" <- 1.04 ("initH")
          "vcount" <- w927
          "hbias" <- w924
          "hcount" <- w927
          "heading error" <- w924
          "pos error" <- w924
          "Kalmann init" <- TRUE ("POS init")
          "get map name" <- TRUE
        }
        frame #1 {
          n571 = disable-structure shown="Enabled" {
            disable-tunnel: w935 -> [w1045 _]
            frame Enabled {
              n572 = node-c288(i64 10 ("Period")) -> (w1044:T2)  [unwired: 3 in]
              n573 = timed-loop {
                shift-right: [w1046] -> _
                shift-left: w1045 -> [w1047]
                timing: w1044 -> [_]
                timing-out: [_] -> w1043
                stop <- FALSE stop-if-true
                n574 = node-c288() -> ()  [unwired: 1 in]
                n575 = flat-sequence {
                  tunnel: [w1063] -> w1049
                  tunnel: w1047 -> [w1063]
                  tunnel: w1049 -> [w1066]
                  tunnel: [w1065] -> w1048
                  tunnel: [w1380] -> w1046
                  tunnel: w1048 -> [w1380]
                  frame #0 {
                    n576 = call "Tick Count"() -> ("Tick Count(uSec)"=w1060:u32)
                    n577 = global read "rio_Global.vi" "C_yaw_rate"() -> (w1055:dbl)
                    n578 = global read "rio_Global.vi" "C_VS_CAN"() -> (→"VS_CAN":dbl)
                    n579 = feedback-in #2(w1060) -> ()
                    n580 = feedback #2(w1060) -> (w1061:u32)
                    n581 = Subtract(x=w1060, y=w1061) -> (x-y=w1059:u32)
                    n582 = Subtract(x=w1055, y=0.25) -> (x-y=→"yaw_rate":dbl)
                    n583 = To Double Precision Float(number=w1059) -> (double precision float=w1058:dbl)
                    n584 = Multiply(x=w1058, y=1e-06) -> (x*y=→"dt":dbl)
                  }
                  frame #1 {
                    n585 = flat-sequence {
                      tunnel: w1066 -> [w1109]
                      tunnel: [w1109] -> w1064
                      tunnel: [w1134] -> w1065
                      tunnel: w1064 -> [w1135]
                      frame #0 {
                        n586 = global read "rio_Global.vi" "gps_pos 1"() -> (w1106:dbl[])
                        "pos_gps" <- w1106
                        n587 = global read "rio_Global.vi" "gps_vel 1"() -> (w1093:dbl[])
                        n588 = local read "VS_CAN"() -> (w1072:dbl)
                        n589 = local read "VS_CAN"() -> (w1071:dbl)
                        n590 = local read "VS_CAN"() -> (w1073:dbl)
                        n591 = Equal To 0?(x=w1072) -> (x = 0?=w1074:bool)
                        n592 = Index Array(array=w1106, index #1=0 ("index")) -> (element #1=w1103:dbl, element #2=w1102:dbl, element #3=w1067:dbl)  [unwired: 2 in]
                        n593 = Index Array(array=w1093, index #1=0 ("index"), index #2=1 ("index"), index #3=4 ("index"), index #4=2 ("index")) -> (element #1=w1076:dbl, element #2=w1089:dbl, element #3=w1086:dbl, element #4=w1078:dbl)
                        n594 = Not Equal To 0?(x=w1102) -> (x != 0?=w1099:bool)
                        n595 = Greater Or Equal To 0?(x=w1071) -> (x >= 0?=w1095:bool)
                        n596 = feedback #3(w1103) -> (w1101:dbl)
                        n597 = feedback-in #3(w1103) -> ()
                        n598 = case shown="True" w1074 {
                          frame False {
                          }
                          frame True {
                            w1113 = u64 18446744073709551615
                            n599 = local read "hcount"() -> (w1116:u64)
                            n600 = local read "hbias"() -> (w1119:dbl)
                            n601 = Increment(x=w1116) -> (x+1=w1115:u64)
                            n602 = local read "yaw_rate"() -> (w1110:dbl)
                            n603 = Not Equal?(x=w1116, y=w1113) -> (x != y?=w1114:bool)
                            n604 = Multiply(x=w1119, y=w1116) -> (x*y=w1118:dbl)
                            n605 = Add(x=w1110, y=w1118) -> (x+y=w1117:dbl)
                            n606 = Select(t=w1115, s=w1114, f=w1113) -> (s? t:f=w1112:u64)
                            n607 = Divide(x=w1117, y=w1112) -> (x/y=w1111:dbl)
                            n608 = local write "hcount"(w1112) -> ()
                            n609 = local write "hbias"(w1111) -> ()
                          }
                        }
                        n610 = Absolute Value(x=w1073) -> (abs(x)=w1079:dbl)
                        n611 = call "Convert to Dynamic Data2"("Double"=w1067) -> ("Dynamic Data Type"=→"Waveform Chart 2":dynamicdata)  [unwired: 3 in]
                        n612 = Greater?(x=w1103, y=w1101) -> (0:w1100:bool)
                        n613 = feedback #4(w1076) -> (w1085:dbl)
                        n614 = feedback-in #4(w1076) -> ()
                        n615 = call "angleconv.vi"("deg"=w1086) -> ("rad"=w1077:dbl)  [unwired: 9 in, 1 out]
                        n616 = Divide(x=w1078, y=w1079) -> (x/y=w1108:dbl)
                        n617 = Select(t=0.0, s=w1095, f=3.141592653589793) -> (s? t:f=w1094:dbl)
                        n618 = And(x=w1100, y=w1099) -> (x .and. y?=→"get position":bool)
                        n619 = Greater?(x=w1076, y=w1085) -> (0:w1090:bool)
                        n620 = call "headingoperater.vi"("h1"=w1094, "h2"=w1077) -> ("h2-h1"=→"h_gps":dbl)  [unwired: 8 in, 1 out]
                        n621 = Not Equal To 0?(x=w1089) -> (x != 0?=w1088:bool)
                        n622 = Decrement(x=w1108) -> (x-1=w1082:dbl)
                        n623 = Absolute Value(x=w1082) -> (abs(x)=w1083:dbl)
                        n624 = And(x=w1090, y=w1088) -> (x .and. y?=w1069:bool)
                        "get heading" <- w1069
                        n625 = Greater?(x=w1079, y=15.0) -> (0:w1070:bool)
                        n626 = Less?(x=w1083, y=0.05) -> (x < y?=w1075:bool)
                        n627 = Compound Arithmetic op=AND(w1069, w1075, w1070) -> (w1107:bool)
                        n628 = case shown="True" w1107 {
                          tunnel: w1108 -> [_ w1127]
                          frame False {
                          }
                          frame True {
                            w1121 = u64 18446744073709551615
                            n629 = local read "vcount"() -> (w1124:u64)
                            n630 = local read "vgain"() -> (w1129:dbl)
                            n631 = Increment(x=w1124) -> (x+1=w1123:u64)
                            n632 = Multiply(x=w1129, y=w1124) -> (x*y=w1128:dbl)
                            n633 = Not Equal?(x=w1124, y=w1121) -> (x != y?=w1122:bool)
                            n634 = Add(x=w1127, y=w1128) -> (x+y=w1126:dbl)
                            n635 = Select(t=w1123, s=w1122, f=w1121) -> (s? t:f=w1120:u64)
                            n636 = local write "vcount"(w1120) -> ()
                            n637 = Divide(x=w1126, y=w1120) -> (x/y=w1125:dbl)
                            n638 = local write "vgain"(w1125) -> ()
                          }
                        }
                      }
                      frame #1 {
                        n639 = local read "dt"() -> (w1133:dbl)
                        n640 = In Range and Coerce(upper limit=0.05, x=w1133, lower limit=1e-06 ("y")) -> (In Range?=w1130:bool)  [unwired: 1 out]
                        n641 = case shown="True" w1130 {
                          tunnel: w1135 -> [w1136 w1139]
                          tunnel: [w1136 w1138] -> w1134
                          frame False {
                          }
                          frame True {
                            n642 = flat-sequence {
                              tunnel: w1139 -> [w1179]
                              tunnel: [w1158] -> w1137
                              tunnel: [w1207] -> w1138
                              tunnel: w1137 -> [w1185]
                              frame #0 {
                                n643 = local read "yaw_rate"() -> (w1146:dbl)
                                n644 = local read "hbias"() -> (w1147:dbl)
                                n645 = local read "VS_CAN"() -> (w1150:dbl)
                                n646 = local read "VS_CAN"() -> (w1149:dbl)
                                n647 = Subtract(x=w1146, y=w1147) -> (x-y=w1144:dbl)
                                n648 = local read "vgain"() -> (w1154:dbl)
                                n649 = Equal To 0?(x=w1149) -> (x = 0?=w1145:bool)
                                n650 = Negate(x=w1144) -> (-x=w1141:dbl)
                                n651 = Multiply(x=w1150, y=w1154) -> (x*y=w1153:dbl)
                                n652 = Select(t=0.0, s=w1145, f=w1141) -> (s? t:f=w1143:dbl)
                                n653 = call "angleconv.vi"("deg"=w1143) -> ("rad"=w1151:dbl)  [unwired: 9 in, 1 out]
                                n654 = Divide(x=w1153, y=3.6) -> (x/y=w1152:dbl)
                                n655 = Index Array(array=w1179, index #1=0 ("index"), index #2=3 ("index"), index #3=1 ("index"), index #4=3 ("index")) -> (element #1=w1173:dbl, element #2=w1172:dbl, element #3=w1168:dbl, element #4=w1163:dbl)
                                n656 = local read "dt"() -> (w1176:dbl)
                                n657 = local read "dt"() -> (w1161:dbl)
                                n658 = Multiply(x=w1152, y=w1176) -> (x*y=w1140:dbl)
                                n659 = Multiply(x=w1161, y=w1151) -> (x*y=w1148:dbl)
                                "rt" <- w1148
                                n660 = Cosine(x=w1172) -> (cos(x)=w1177:dbl)
                                n661 = Sine(x=w1172) -> (sin(x)=w1171:dbl)
                                n662 = Multiply(x=w1177, y=w1140) -> (x*y=w1174:dbl)
                                n663 = Multiply(x=w1140, y=w1171) -> (x*y=w1170:dbl)
                                n664 = Add(x=w1173, y=w1174) -> (x+y=w1167:dbl)
                                n665 = Add(x=w1170, y=w1168) -> (x+y=w1166:dbl)
                                n666 = call "headingoperater.vi"("h1"=w1148, "h2"=w1163) -> ("h2+h1"=w1162:dbl)  [unwired: 8 in, 1 out]
                                n667 = Build Array(w1167, w1166, w1152, w1162, w1151) -> (w1158:dbl[])
                                n668 = Index Array(array=w1158, index=3) -> (element=w1157:dbl)
                                n669 = local read "h_gps"() -> (w1156:dbl)
                                n670 = call "headingoperater.vi"("h1"=w1157, "h2"=w1156) -> ("h2-h1"=w1160:dbl)  [unwired: 8 in, 1 out]
                                n671 = Absolute Value(x=w1160) -> (abs(x)=w1155:dbl)
                                n672 = local write "heading error"(w1155) -> ()
                              }
                              frame #1 {
                                n673 = Array Subset(array=w1185, index=0, length=2) -> (w1192:dbl[])
                                n674 = local read "pos_gps"() -> (w1188:dbl[])
                                n675 = local read "Kalmann init"() -> (w1200:bool)
                                n676 = local read "get heading"() -> (w1213:bool)
                                n677 = local read "get position"() -> (w1212:bool)
                                n678 = Array Subset(array=w1188, index=2, length=2) -> (w1191:dbl[])
                                n679 = Subtract(x=w1191, y=w1192) -> (x-y=w1193:dbl[])
                                n680 = case shown="True" w1200 {
                                tunnel: w1213 -> [w1216 w1223]
                                tunnel: w1212 -> [w1220 w1222]
                                tunnel: [w1214 w1221] -> w1209
                                frame False {
                                n681 = local read "heading error"() -> (w1217:dbl)
                                n682 = Less?(x=w1217, y=0.05) -> (x < y?=w1218:bool)
                                n683 = And(x=w1216, y=w1218) -> (x .and. y?=w1215:bool)
                                n684 = Or(x=w1215, y=w1220) -> (x .or. y?=w1214:bool)
                                }
                                frame True {
                                n685 = disable-structure shown="Enabled" {
                                disable-tunnel: w1223 -> [w1226 w1228]
                                disable-tunnel: w1222 -> [w1225 w1227]
                                disable-tunnel: [w1224 w1229] -> w1221
                                frame Disabled {
                                n686 = And(x=w1226, y=w1225) -> (x .and. y?=w1224:bool)
                                }
                                frame Enabled {
                                n687 = Or(x=w1228, y=w1227) -> (x .or. y?=w1229:bool)
                                }
                                }
                                }
                                }
                                n688 = Square(x=w1193) -> (x^2=w1194:dbl[])
                                n689 = Add Array Elements(numeric array=w1194) -> (sum=w1195:dbl)
                                n690 = Square Root(x=w1195) -> (sqrt(x)=w1184:dbl)
                                n691 = local read "VS_CAN"() -> (w1196:dbl)
                                n692 = local read "heading error"() -> (w1203:dbl)
                                n693 = local read "Kalmann init"() -> (w1201:bool)
                                n694 = Absolute Value(x=w1196) -> (abs(x)=w1211:dbl)
                                n695 = Greater?(x=w1211, y=5.0) -> (0:w1208:bool)
                                n696 = Less?(x=w1203, y=1.0) -> (x < y?=w1202:bool)
                                n697 = Or(x=w1202, y=w1201) -> (x .or. y?=w1204:bool)
                                n698 = And(x=w1209, y=w1208) -> (x .and. y?=w1205:bool)
                                n699 = And(x=w1205, y=w1204) -> (x .and. y?=w1198:bool)
                                n700 = Less?(x=w1184, y=50.0) -> (x < y?=w1181:bool)
                                n701 = Select(t=FALSE, s="GPS init", f=w1198) -> (s? t:f=w1182:bool)
                                n702 = And(x=w1182, y=w1181) -> (x .and. y?=w1180:bool)
                                n703 = case shown="True" w1180 {
                                tunnel: [w1235 w1262] -> w1207
                                tunnel: w1185 -> [w1230 w1265]
                                frame False {
                                n704 = local read "VS_CAN"() -> (w1231:dbl)
                                n705 = local read "Kalmann init"() -> (w1237:bool)
                                n706 = Equal To 0?(x=w1231) -> (x = 0?=w1236:bool)
                                n707 = local read "GPS init"() -> (w1232:bool)
                                n708 = And(x=w1237, y=w1236) -> (x .and. y?=w1234:bool)
                                n709 = Or(x=w1234, y=w1232) -> (x .or. y?=w1233:bool)
                                n710 = case shown="False" w1233 {
                                tunnel: w1230 -> [w1238 w1239]
                                tunnel: [w1238 w1241] -> w1235
                                tunnel: w1232 -> [_ w1240]
                                frame False {
                                }
                                frame True {
                                n711 = case shown="True" w1240 {
                                tunnel: [w1252 w1261] -> w1241
                                tunnel: w1239 -> [w1247 w1255]
                                frame True {
                                n712 = Index Array(array=w1247, index #1=2 ("index")) -> (element #2=w1242:dbl, element #3=w1245:dbl)  [unwired: 2 in, 1 out]
                                n713 = local read "pos_gps"() -> (w1248:dbl[])
                                n714 = local write "GPS init"(FALSE ("GPS init")) -> ()
                                n715 = Index Array(array=w1248, index #1=2 ("index")) -> (element #1=w1250:dbl, element #2=w1249:dbl)  [unwired: 1 in]
                                n716 = local read "h_gps"() -> (w1243:dbl)
                                n717 = Build Array(w1250, w1249, w1242, w1243, w1245) -> (w1252:dbl[])
                                }
                                frame False {
                                w1254 = 0.0 ("element")
                                n718 = Index Array(array=w1255, index=3) -> (element=w1253:dbl)
                                n719 = local read "pos_gps"() -> (w1257:dbl[])
                                n720 = Index Array(array=w1257, index #1=2 ("index")) -> (element #1=w1259:dbl, element #2=w1258:dbl)  [unwired: 1 in]
                                n721 = Build Array(w1259, w1258, w1254, w1253, w1254) -> (w1261:dbl[])
                                }
                                }
                                }
                                }
                                }
                                frame True {
                                n722 = flat-sequence {
                                tunnel: w1265 -> [w1266]
                                tunnel: [w1266] -> w1264
                                tunnel: w1264 -> [w1307]
                                tunnel: [w1307] -> w1263
                                tunnel: w1263 -> [w1351]
                                tunnel: [w1354] -> w1262
                                frame #0 {
                                w1275 = 0.0 ("element")
                                w1279 = 0.0 ("element")
                                w1281 = 0.0 ("element")
                                w1283 = 0.0 ("element")
                                w1285 = 0.0 ("element")
                                n723 = Index Array(array=w1266, index #1=3 ("index"), index #2=2 ("index"), index #3=3 ("index"), index #4=2 ("index")) -> (element #1=w1295:dbl, element #2=w1297:dbl, element #3=w1300:dbl, element #4=w1289:dbl)
                                n724 = Negate(x=w1297) -> (-x=w1296:dbl)
                                n725 = Sine & Cosine(0:w1300) -> (1:w1292:dbl, 2:w1290:dbl)
                                n726 = Multiply(x=w1296, y=w1292) -> (x*y=w1293:dbl)
                                n727 = Multiply(x=w1290, y=w1289) -> (x*y=w1288:dbl)
                                n728 = Cosine(x=w1295) -> (cos(x)=w1294:dbl)
                                n729 = Build Array(w1285, w1285, w1294, w1293, 0.0 ("element")) -> (w1287:dbl[])
                                n730 = Build Array(w1283, w1283, w1292, w1288, 0.0 ("element")) -> (w1286:dbl[])
                                n731 = Build Array(w1281, w1281, w1281, w1281, w1281) -> (w1280:dbl[])
                                n732 = Build Array(w1279, w1279, w1279, w1279, 1.0 ("element")) -> (w1277:dbl[])
                                n733 = Build Array(w1275, w1275, w1275, w1275, w1275) -> (w1276:dbl[])
                                n734 = Build Array(w1287, w1286, w1280, w1277, w1276) -> (w1273:dbl[][])
                                n735 = call-poly <vilib>:"Array To Matrix.vi"("Real 2D Array"=w1273) -> ("Real Matrix"=w1271:T29)
                                n736 = global read "rio_Global.vi" "P"() -> (w1274:T29)
                                n737 = Transpose Matrix(1:w1271) -> (0:w1270:T29)
                                n738 = call-poly <vilib>:"Multiply.vi"("Real Matrix B"=w1274, "Real Matrix A"=w1271) -> ("A * B"=w1272:T29)
                                n739 = call-poly <vilib>:"Multiply.vi"("Real Matrix B"=w1270, "Real Matrix A"=w1272) -> ("A * B"=w1269:T29)
                                n740 = global read "rio_Global.vi" "Q"() -> (w1268:T29)
                                n741 = call-poly <vilib>:"Add.vi"("Real Matrix B"=w1268, "Real Matrix A"=w1269) -> ("A + B"=w1267:T29)
                                n742 = global write "rio_Global.vi" "Pp"(w1267) -> ()
                                }
                                frame #1 {
                                n743 = global read "rio_Global.vi" "Pp"() -> (w1332:T29)
                                n744 = global read "rio_Global.vi" "H"() -> (w1331:T29)
                                n745 = Array Subset(array=w1307, index=0, length=2) -> (w1314:dbl[])
                                n746 = local read "pos_gps"() -> (w1310:dbl[])
                                n747 = call-poly <vilib>:"Multiply.vi"("Real Matrix B"=w1332, "Real Matrix A"=w1331) -> ("A * B"=w1330:T29)
                                n748 = Transpose Matrix(1:w1331) -> (0:w1329:T29)
                                n749 = call-poly <vilib>:"Multiply.vi"("Real Matrix B"=w1329, "Real Matrix A"=w1330) -> ("A * B"=w1328:T29)
                                n750 = Array Subset(array=w1310, index=2, length=2) -> (w1313:dbl[])
                                n751 = Subtract(x=w1313, y=w1314) -> (x-y=w1315:dbl[])
                                n752 = global read "rio_Global.vi" "H"() -> (w1326:T29)
                                n753 = global read "rio_Global.vi" "R"() -> (w1327:T29)
                                n754 = global read "rio_Global.vi" "Pp"() -> (w1325:T29)
                                n755 = call-poly <vilib>:"Add.vi"("Real Matrix B"=w1327, "Real Matrix A"=w1328) -> ("A + B"=w1322:T29)
                                n756 = Square(x=w1315) -> (x^2=w1316:dbl[])
                                n757 = Transpose Matrix(1:w1326) -> (0:w1324:T29)
                                n758 = local read "heading error"() -> (w1319:dbl)
                                n759 = call-poly <vilib>:"Multiply.vi"("Real Matrix B"=w1324, "Real Matrix A"=w1325) -> ("A * B"=w1323:T29)
                                n760 = Add Array Elements(numeric array=w1316) -> (sum=w1317:dbl)
                                n761 = call-poly <vilib>:"Inverse Matrix.vi"("Input Matrix"=w1322) -> ("Inverse Matrix"=w1321:T29)  [unwired: 1 in, 1 out]
                                n762 = call-poly <vilib>:"Multiply.vi"("Real Matrix B"=w1321, "Real Matrix A"=w1323) -> ("A * B"=w1320:T29)
                                n763 = Square Root(x=w1317) -> (sqrt(x)=w1302:dbl)
                                n764 = global write "rio_Global.vi" "K"(w1320) -> ()
                                n765 = local write "pos error"(w1302) -> ()
                                n766 = Less?(x=w1302, y=2.5) -> (x < y?=w1304:bool)
                                n767 = Less?(x=w1319, y=0.05) -> (x < y?=w1305:bool)
                                n768 = And(x=w1305, y=w1304) -> (x .and. y?=w1303:bool)
                                n769 = case shown="True" w1303 {
                                frame False {
                                }
                                frame True {
                                n770 = local write "Kalmann init"(FALSE ("Kalman init")) -> ()
                                }
                                }
                                }
                                frame #2 {
                                n771 = disable-structure shown="Enabled" {
                                disable-tunnel: [w1366 w1367] -> w1353
                                frame Disabled {
                                n772 = local read "get heading"() -> (w1366:bool)
                                }
                                frame Enabled {
                                n773 = local read "heading error"() -> (w1370:dbl)
                                n774 = local read "Kalmann init"() -> (w1368:bool)
                                n775 = Less?(x=w1370, y=0.1) -> (x < y?=w1369:bool)
                                n776 = Or(x=w1369, y=w1368) -> (x .or. y?=w1367:bool)
                                }
                                }
                                n777 = Index Array(array=w1351, index=3) -> (element=w1357:dbl)
                                n778 = global read "rio_Global.vi" "K"() -> (w1365:T29)
                                n779 = global read "rio_Global.vi" "H"() -> (w1364:T29)
                                n780 = global read "rio_Global.vi" "Pp"() -> (w1362:T29)
                                n781 = call-poly <vilib>:"Multiply.vi"("Real Matrix B"=w1364, "Real Matrix A"=w1365) -> ("A * B"=w1363:T29)
                                n782 = global read "rio_Global.vi" "Pp"() -> (w1360:T29)
                                n783 = call-poly <vilib>:"Multiply.vi"("Real Matrix B"=w1362, "Real Matrix A"=w1363) -> ("A * B"=w1361:T29)
                                n784 = call-poly <vilib>:"Subtract.vi"("Real Matrix B"=w1361, "Real Matrix A"=w1360) -> ("A - B"=w1359:T29)
                                n785 = global write "rio_Global.vi" "P"(w1359) -> ()
                                n786 = case shown="True" w1353 {
                                tunnel: w1357 -> [w1372 w1379]
                                tunnel: [w1372 w1374] -> w1352
                                frame False {
                                }
                                frame True {
                                n787 = global read "rio_Global.vi" "K"() -> (w1378:T29)
                                n788 = Index Array(array=w1378, index (row)=3, index (col)=2 ("disabled index (col)")) -> (element=w1375:dbl)
                                n789 = local read "h_gps"() -> (w1373:dbl)
                                n790 = call "headingweightsum2.vi"("a"=w1375, "h2"=w1373, "h1"=w1379) -> ("a*h2+(1-a)*h1"=w1374:dbl)  [unwired: 8 in]
                                }
                                }
                                n791 = local read "pos_gps"() -> (w1337:dbl[])
                                n792 = call-poly <vilib>:"Array To Matrix.vi"("Real 1D Array"=w1351) -> ("Real Matrix (Column Vector)"=w1345:T29)
                                n793 = Array Subset(array=w1337, index=2, length=2) -> (w1338:dbl[])
                                n794 = Build Array (concatenate)(w1338, w1352) -> (w1334:dbl[])
                                n795 = global read "rio_Global.vi" "H"() -> (w1350:T29)
                                n796 = call-poly <vilib>:"Multiply.vi"("Real Matrix B"=w1345, "Real Matrix A"=w1350) -> ("A * B"=w1349:T29)
                                n797 = call-poly <vilib>:"Array To Matrix.vi"("Real 1D Array"=w1334) -> ("Real Matrix (Column Vector)"=w1348:T29)
                                n798 = call-poly <vilib>:"Subtract.vi"("Real Matrix B"=w1349, "Real Matrix A"=w1348) -> ("A - B"=w1346:T29)
                                n799 = global read "rio_Global.vi" "K"() -> (w1347:T29)
                                n800 = call-poly <vilib>:"Multiply.vi"("Real Matrix B"=w1346, "Real Matrix A"=w1347) -> ("A * B"=w1341:T29)
                                n801 = call-poly <vilib>:"Multiply.vi"("Real Matrix A"=w1341, "Real Scalar c"=0.7) -> ("c * A"=w1339:T29)
                                n802 = call-poly <vilib>:"Add.vi"("Real Matrix B"=w1345, "Real Matrix A"=w1339) -> ("A + B"=w1344:T29)
                                n803 = call-poly <vilib>:"Matrix To Array.vi"("Real Matrix"=w1344) -> ("Real 2D Array"=w1343:dbl[][])
                                n804 = Index Array(array=w1343, index (col)=0 ("disabled index (col)")) -> (element=w1356:dbl[])  [unwired: 1 in]
                                n805 = Replace Array Subset(array=w1356, new element=w1352, index=3) -> (w1354:dbl[])
                                }
                                }
                                }
                                }
                              }
                            }
                          }
                        }
                      }
                    }
                  }
                  frame #2 {
                    n806 = local read "h_gps"() -> (w1386:dbl)
                    n807 = local read "dt"() -> (w1383:dbl)
                    n808 = Index Array(array=w1380, index=3) -> (element=w1390:dbl)
                    n809 = Array Subset(array=w1380, index=0, length=2) -> (→"pos":dbl[])
                    n810 = Greater Than 0?(x=w1383) -> (x > 0?=w1382:bool)
                    n811 = call "angleconv.vi"("rad"=w1390) -> ("deg"=→"Heading":dbl)  [unwired: 9 in, 1 out]
                    n812 = Greater?(x=1.0, y=w1383) -> (0:w1385:bool)
                    n813 = call "headingoperater.vi"("h1"=0.0, "h2"=w1386) -> ("h2+h1"=w1387:dbl)  [unwired: 8 in, 1 out]
                    n814 = call "angleconv.vi"("rad"=w1387) -> ("deg"=→"H_GPS":dbl)  [unwired: 9 in, 1 out]
                    n815 = Compound Arithmetic op=AND(w1385, w1382) -> (w1381:bool)
                    n816 = case shown="True" w1381 {
                      tunnel: w1380 -> [_ w1396]
                      frame False {
                      }
                      frame True {
                        n817 = flat-sequence {
                          tunnel: w1396 -> [w1420]
                          frame #0 {
                            n818 = Get Date/Time In Seconds() -> (seconds since 1Jan1904=w1411:timestamp)
                            n819 = To Double Precision Float(number=w1411) -> (double precision float=w1405:dbl)
                            n820 = global read "rio_Global.vi" "LCM_POS_T"() -> (w1419:T30)
                            n821 = local read "Kalmann init"() -> (w1401:bool)
                            n822 = Unbundle By Name(w1419) -> ("hash"=w1416:i64)
                            n823 = local read "dt"() -> (w1400:dbl)
                            n824 = Multiply(x=w1405, y=1000000.0) -> (x*y=w1403:dbl)
                            n825 = Array To Cluster(array=w1420) -> (cluster=w1418:T31)
                            n826 = Select(t=0.0, s=w1401, f=w1400) -> (s? t:f=w1398:dbl)
                            n827 = call "hash.vi"("input"=w1416) -> ("output"=w1415:i64)  [unwired: 10 in]
                            n828 = To Quad Integer(1:w1403) -> (0:w1402:i64)
                            n829 = Unbundle(w1418) -> ("Real 2D Array[0]"=w1410:dbl, "Real 2D Array[1]"=w1409:dbl, "Real 2D Array[2]"=w1408:dbl, "Real 2D Array[3]"=w1407:dbl, "Real 2D Array[4]"=w1406:dbl)
                            n830 = Bundle(cluster=w1419, "hash"=w1415, "sys time"=w1402, "dt"=w1398, "x"=w1410, "y"=w1409, "speed"=w1408, "heading"=w1407, "yaw_rate"=w1406) -> (w1397:T30)
                            n831 = Flatten To String(anything=w1397, prepend array or string size? (T)=FALSE) -> (data string=w1413:string)  [unwired: 2 in, 2 out]
                            n832 = global read "rio_Global.vi" "LCM"() -> (w1412:T9)
                            n833 = call "LCM_send.vi"("DATA"=w1413, "ID"="POS_T", "LCM"=w1412) -> ()  [unwired: 7 in, 2 out]
                          }
                        }
                      }
                    }
                  }
                }
                n834 = node-c288() -> ()  [unwired: 1 in, 1 out]
              }
              n835 = node-c288(w1043) -> ()  [unwired: 1 out]
            }
            frame Disabled {
            }
          }
          n836 = while {
            shift-right: [w1040] -> w931
            shift-left: refnum<visa-resource-name> "ASRL3::INSTR" ("VISA resource name") -> [w1041]
            stop <- w1039 continue-if-true
            n837 = VISA Open(VISA resource name=w1041) -> (VISA resource name=w1040:refnum<visa-resource-name>, error out=w1039:errorcluster)  [unwired: 4 in]
          }
          n838 = VISA Clear(VISA resource name=w931) -> (VISA resource name out=w933:refnum<visa-resource-name>)  [unwired: 1 in, 1 out]
          n839 = property class="Instr"(reference=w933, "General Settings:Timeout Value"=u32 10) -> (reference out=w934:refnum<visa-resource-name>)  [unwired: 1 in, 1 out]
          n840 = while {
            tunnel: w934 -> [w938]
            stop <- FALSE stop-if-true
            n841 = property class="Instr"(reference=w938) -> (reference out=w937:refnum<visa-resource-name>, "Bytes at Port"=w936:u32)  [unwired: 1 in, 1 out]
            n842 = case shown="1, Default" w936 {
              selector: w936 -> [_ w944]
              tunnel: w937 -> [_ w945]
              frame 0 {
                n843 = Wait (ms)(milliseconds to wait=u32 10) -> ()  [unwired: 1 out]
              }
              frame 1, Default {
                n844 = VISA Read(VISA resource name=w945, byte count=w944) -> (read buffer=w946:string)  [unwired: 1 in, 3 out]
                "read buffer" <- w946
                n845 = local read "ecef ref"() -> (w941:dbl[])
                n846 = call "nmea.vi"("ecef ref"=w941, "NMEA"=w946) -> ("output"=w943:dbl[], "type"=w942:u32)  [unwired: 8 in]
                n847 = case shown="1" w942 {
                  tunnel: w943 -> [_ w952 w1014]
                  frame 0, Default {
                  }
                  frame 1 {
                    n848 = Index Array(array=w952, index=1) -> (element=w950:dbl)
                    n849 = Not Equal To 0?(x=w950) -> (x != 0?=w949:bool)
                    n850 = local read "get map name"() -> (w948:bool)
                    n851 = And(x=w949, y=w948) -> (x .and. y?=w947:bool)
                    n852 = case shown="True" w947 {
                      tunnel: w952 -> [w953 w1010]
                      frame False {
                        n853 = global write "rio_Global.vi" "gps_pos 1"(w953) -> ()
                        n854 = disable-structure shown="Enabled" {
                          disable-tunnel: w953 -> [w955 _]
                          frame Enabled {
                            n855 = Index Array(array=w955, index=1) -> (element=w957:dbl)
                            n856 = Not Equal To 0?(x=w957) -> (x != 0?=w954:bool)
                            n857 = case shown="True" w954 {
                              tunnel: w955 -> [_ w977]
                              frame False {
                              }
                              frame True {
                                n858 = Get Date/Time In Seconds() -> (seconds since 1Jan1904=w962:timestamp)
                                n859 = To Double Precision Float(number=w962) -> (double precision float=w961:dbl)
                                n860 = global read "rio_Global.vi" "LCM_GGA_T"() -> (w986:T32)
                                n861 = Array To Cluster(array=w977) -> (cluster=w985:T33)
                                n862 = Unbundle By Name(w986) -> ("hash"=w982:i64)
                                n863 = Multiply(x=w961, y=1000000.0) -> (x*y=w959:dbl)
                                n864 = Unbundle(w985) -> ("output[0]"=w987:dbl, "output[2]"=w976:dbl, "output[3]"=w975:dbl, "output[4]"=w974:dbl, "output[6]"=w973:dbl, "output[7]"=w971:dbl, "output[8]"=w969:dbl, "output[9]"=w967:dbl, "output[12]"=w966:dbl, "output[13]"=w965:dbl, "output[14]"=w964:dbl)  [unwired: 4 out]
                                n865 = local read "map name"() -> (w963:T1)
                                n866 = call "hash.vi"("input"=w982) -> ("output"=w981:i64)  [unwired: 10 in]
                                n867 = To Quad Integer(1:w959) -> (0:w958:i64)
                                n868 = To Long Integer(number=w973) -> (32bit integer=w972:i32)
                                n869 = To Long Integer(number=w971) -> (32bit integer=w970:i32)
                                n870 = To Long Integer(number=w969) -> (32bit integer=w968:i32)
                                n871 = Bundle(cluster=w986, "hash"=w981, "sys time"=w958, "time"=w987, "x"=w976, "y"=w975, "h"=w974, "numSV"=w972, "postype"=w970, "lag"=w968, "hordev"=w967, "lat"=w966, "lon"=w965, "hgt"=w964, "map_idx"=w963) -> (w983:T32)
                                n872 = Flatten To String(anything=w983, prepend array or string size? (T)=FALSE) -> (data string=w979:string)  [unwired: 2 in, 2 out]
                                n873 = global read "rio_Global.vi" "LCM"() -> (w978:T9)
                                n874 = call "LCM_send.vi"("DATA"=w979, "ID"="GGA_1", "LCM"=w978) -> ()  [unwired: 7 in, 2 out]
                              }
                            }
                          }
                          frame Disabled {
                          }
                        }
                      }
                      frame True {
                        n875 = local write "get map name"(FALSE ("get map name")) -> ()
                        n876 = Index Array(array=w1010, index #1=12 ("index")) -> (element #1=w1005:dbl, element #2=w1001:dbl)  [unwired: 1 in]
                        n877 = for {
                          N: 11 -> [_]
                          tunnel: [w1012] -> w999 mode=indexing
                          tunnel: [w1011] -> w997 mode=indexing
                          i -> [w1013]
                          n878 = call "getecefdcmref.vi"("map name"=w1013) -> ("lat"=w1012:dbl, "lon"=w1011:dbl)  [unwired: 10 in, 3 out]
                        }
                        n879 = Multiply(x=w1005, y=3.141592653589793) -> (x*y=w1007:dbl)
                        n880 = Multiply(x=w1001, y=3.141592653589793) -> (x*y=w1003:dbl)
                        n881 = Divide(x=w1007, y=180.0) -> (x/y=w998:dbl)
                        n882 = Divide(x=w1003, y=180.0) -> (x/y=w996:dbl)
                        n883 = Subtract(x=w999, y=w998) -> (x-y=w995:dbl[])
                        n884 = Subtract(x=w997, y=w996) -> (x-y=w994:dbl[])
                        n885 = Square(x=w995) -> (x^2=w993:dbl[])
                        n886 = Square(x=w994) -> (x^2=w992:dbl[])
                        n887 = Add(x=w993, y=w992) -> (x+y=w991:dbl[])
                        n888 = Array Max & Min(array=w991) -> (min index (indices)=w990:i32)  [unwired: 3 out]
                        "map name" <- w990
                        n889 = call "getecefdcmref.vi"("map name"=w990) -> ("XYZ"=→"ecef ref":dbl[])  [unwired: 10 in, 4 out]
                      }
                    }
                  }
                  frame 2 {
                    n890 = global write "rio_Global.vi" "gps_vel 1"(w1014) -> ()
                    n891 = disable-structure shown="Enabled" {
                      disable-tunnel: w1014 -> [w1018 _]
                      frame Enabled {
                        n892 = Index Array(array=w1018, index=1) -> (element=w1017:dbl)
                        n893 = Not Equal To 0?(x=w1017) -> (x != 0?=w1015:bool)
                        n894 = case shown="True" w1015 {
                          tunnel: w1018 -> [_ w1037]
                          frame False {
                          }
                          frame True {
                            n895 = Get Date/Time In Seconds() -> (seconds since 1Jan1904=w1023:timestamp)
                            n896 = To Double Precision Float(number=w1023) -> (double precision float=w1022:dbl)
                            n897 = global read "rio_Global.vi" "LCM_RMC_T"() -> (w1038:T34)
                            n898 = Unbundle By Name(w1038) -> ("hash"=w1034:i64)
                            n899 = Multiply(x=w1022, y=1000000.0) -> (x*y=w1020:dbl)
                            n900 = Array To Cluster(array=w1037) -> (cluster=w1036:T35)
                            n901 = To Quad Integer(1:w1020) -> (0:w1019:i64)
                            n902 = call "hash.vi"("input"=w1034) -> ("output"=w1033:i64)  [unwired: 10 in]
                            n903 = Unbundle(w1036) -> ("output[0]"=w1028:dbl, "output[2]"=w1027:dbl, "output[4]"=w1026:dbl, "output[5]"=w1025:dbl, "output[6]"=w1024:dbl)  [unwired: 2 out]
                            n904 = Bundle(cluster=w1038, "hash"=w1033, "sys time"=w1019, "time"=w1028, "speed"=w1027, "heading"=w1026, "lat"=w1025, "lon"=w1024) -> (w1029:T34)
                            n905 = Flatten To String(anything=w1029, prepend array or string size? (T)=FALSE) -> (data string=w1031:string)  [unwired: 2 in, 2 out]
                            n906 = global read "rio_Global.vi" "LCM"() -> (w1030:T9)
                            n907 = call "LCM_send.vi"("DATA"=w1031, "ID"="RMC_1", "LCM"=w1030) -> ()  [unwired: 7 in, 2 out]
                          }
                        }
                      }
                      frame Disabled {
                      }
                    }
                  }
                }
              }
            }
          }
        }
      }
    }
    frame Disabled {
    }
  }
  n908 = flat-sequence {
    tunnel: [w1425] -> w1
    tunnel: w1 -> [w1432]
    frame #0 {
      n909 = for {
        N: 257 -> [_]
        tunnel: [w1431] -> w1429 mode=indexing
        i -> [w1431]
      }
      n910 = Multiply(x=w1429, y=0.5) -> (x*y=w1425:dbl[])
      n911 = global write "rio_Global.vi" "x_view 2"(w1425) -> ()
      n912 = Array Subset(array=w1425, index=30) -> (w1426:dbl[])  [unwired: 1 in]
      n913 = global write "rio_Global.vi" "x_view"(w1426) -> ()
    }
    frame #1 {
      n914 = while {
        tunnel: w1432 -> [w1433]
        stop <- FALSE stop-if-true
        n915 = flat-sequence {
          tunnel: [w1436] -> w1434
          tunnel: w1433 -> [w1436]
          tunnel: w1434 -> [w1438]
          frame #0 {
            n916 = Wait Until Next ms Multiple(millisecond multiple=u32 33) -> ()  [unwired: 1 out]
          }
          frame #1 {
            n917 = call "mobileye_disp.vi"("x_view"=w1438) -> ("XY Graph"=→"XY Graph":cluster{"Y":dbl[], "Y":dbl[]}[])  [unwired: 10 in]
          }
        }
      }
    }
  }
